vi "RTSA_FM_Demodulation.vi"() -> ()   [LabVIEW 2020]
uses:
  <vilib>/sound2/lvsound2.llb/Sound Data Format.ctl
  <vilib>/sound2/lvsound2.llb/Sampling Mode.ctl
  Controls/FIR_Config.ctl
  <vilib>/Analysis/3filter.llb/Filter Passband Type.ctl
  <vilib>/Analysis/4window.llb/windowTd.ctl
  <vilib>/Ngene/CuLab - GPU Accelerated Toolkit/Toolkit/Low_Level/Tensor_Classes/T_Children/T1D/T1D_Children/T1D_SGL/Pull.vi
  <vilib>/Ngene/CuLab - GPU Accelerated Toolkit/Toolkit/Low_Level/Tensor_Classes/T_Children/T2D/T2D_Children/T2D_I16/Pull.vi
  3a16d78b-71d0-4033-90dd-1ad3df79cfc2.vi
  0dbdd736-41c7-4217-8948-0a4463f0bf22.vi
  <vilib>/Ngene/CuLab - GPU Accelerated Toolkit/Toolkit/Low_Level/GPU_Wrapper/cudart/Memory/PULL/1D/cudart_PULL_Data(SGL_1D).vi
  <vilib>/Ngene/CuLab - GPU Accelerated Toolkit/Toolkit/Low_Level/GPU_Wrapper/cudart/Memory/PULL/2D/cudart_PULL_Data(I16_2D).vi
  <extravilib>/ChannelInstances/High Speed Stream-c(dbl,a[.](i8))/_Read For Replicate.vi
  <extravilib>/ChannelInstances/High Speed Stream-a[.](sgl)/_Read For Replicate.vi
  <vilib>/Ngene/CuLab - GPU Accelerated Toolkit/Toolkit/Low_Level/Tensor_Classes/T_Children/T1D/T1D_Children/T1D_I8/T1D_I8.lvclass
  C:/Program Files/National Instruments/LabVIEW 2020/vi.lib/Ngene/CuLab - GPU Accelerated Toolkit/Toolkit/Low_Level/Tensor_Classes/T_Children/T1D/T1D.lvclass
  <vilib>/Ngene/CuLab - GPU Accelerated Toolkit/Toolkit/Low_Level/Tensor_Classes/T_Children/T1D/T1D_Children/T1D_SGL/T1D_SGL.lvclass
  C:/Program Files/National Instruments/LabVIEW 2020/vi.lib/Ngene/CuLab - GPU Accelerated Toolkit/Toolkit/Low_Level/Tensor_Classes/Tensor.lvclass
  <vilib>/Ngene/CuLab - GPU Accelerated Toolkit/Toolkit/Low_Level/Tensor_Classes/T_Children/T2D/T2D_Children/T2D_I16/T2D_I16.lvclass
  C:/Program Files/National Instruments/LabVIEW 2020/vi.lib/Ngene/CuLab - GPU Accelerated Toolkit/Toolkit/Low_Level/Tensor_Classes/T_Children/T2D/T2D.lvclass
  <extravilib>/ChannelInstances/High Speed Stream-c(dbl,a[.](i8))/Instantiate.vi
  <extravilib>/ChannelInstances/High Speed Stream-a[.](sgl)/Instantiate.vi
  <extravilib>/ChannelInstances/High Speed Stream-a[.](sgl)/)Channel.vi
  <extravilib>/ChannelInstances/High Speed Stream-a[.](sgl)/Abort Signal/Init Signal.vi
  <vilib>/sound2/lvsound2.llb/Sound Output Write (DBL Single).vi
  <vilib>/sound2/lvsound2.llb/Sound Output Set Volume (Single).vi
  <extravilib>/ChannelInstances/High Speed Stream-c(dbl,a[.](i8))/)Channel.vi
  <extravilib>/ChannelInstances/High Speed Stream-c(dbl,a[.](i8))/Abort Signal/Init Signal.vi
  <vilib>/Ngene/CuLab - GPU Accelerated Toolkit/Toolkit/Low_Level/Tensor_Classes/T_Children/T1D/T1D_Children/T1D_I8/Push.vi
  <vilib>/Ngene/CuLab - GPU Accelerated Toolkit/Toolkit/API/Numeric/Complex  (API)/Interleaved to Complex/T1D/CU_Interleaved_To_Complex_T1D_CSG.vi
  <vilib>/Ngene/CuLab - GPU Accelerated Toolkit/Toolkit/API/Numeric/Multiply/T1D/CU_MultiplyC_T1D_CSG.vi
  <vilib>/Ngene/CuLab - GPU Accelerated Toolkit/Toolkit/API/Signal Processing/Signal Operation/Digital Down Conversion/CU_Digital_Down_Conversion_T1D_CSG.vi
  <vilib>/Ngene/CuLab - GPU Accelerated Toolkit/Toolkit/API/Signal Processing/Signal Operation/FIR Filter/T1D/CU_FIR_Filter_T1D_CSG.vi
  <vilib>/Ngene/CuLab - GPU Accelerated Toolkit/Toolkit/API/Signal Processing/Signal Operation/Rational Resample/T1D/CU_Rational_Resample_T1D_SGL.vi
  <vilib>/Ngene/CuLab - GPU Accelerated Toolkit/Toolkit/API/Signal Processing/Signal Operation/FIR Filter/T1D/CU_FIR_Filter_T1D_SGL.vi
  <vilib>/Ngene/CuLab - GPU Accelerated Toolkit/Toolkit/Low_Level/Checkers/Check_Tensor_Ref.vi
  <vilib>/Ngene/CuLab - GPU Accelerated Toolkit/Toolkit/Low_Level/Tensor_Classes/Property/Get_Mem_Desc.vi
  <vilib>/Ngene/CuLab - GPU Accelerated Toolkit/Toolkit/Low_Level/Tensor_Classes/T_Children/T1D/Property/Get_Dims.vi
  <vilib>/Ngene/CuLab - GPU Accelerated Toolkit/Toolkit/Low_Level/GPU_Wrapper/cudart/Memory/Utils/cudart_get_type_size(inBytes).vi
  <vilib>/Ngene/CuLab - GPU Accelerated Toolkit/Toolkit/Low_Level/GPU_Wrapper/cudart/cudart_get_Error_String.vi
  <vilib>/Ngene/CuLab - GPU Accelerated Toolkit/Toolkit/Low_Level/Tensor_Classes/T_Children/T2D/Property/Get_Dims.vi
  <vilib>/Analysis/3filter.llb/FIR Filter (CDB).vi
  <vilib>/Analysis/2dsp.llb/Rational Resample (single channel, DBL).vi
  <vilib>/Analysis/3filter.llb/FIR Filter (DBL).vi
  <vilib>/Ngene/CuLab - GPU Accelerated Toolkit/Toolkit/CuLab.lvlib
  <vilib>/ptbypt/NI_PtbyPt.lvlib
  <vilib>/Analysis/NI_AALBase.lvlib
  <vilib>/Analysis/NI_AALPro.lvlib
  <extravilib>/ChannelInstances/High Speed Stream-a[.](sgl).lvlib
  <extravilib>/ChannelInstances/High Speed Stream-c(dbl,a[.](i8)).lvlib
  C:/Program Files/National Instruments/LabVIEW 2020/vi.lib/Ngene/CuLab - GPU Accelerated Toolkit/Toolkit/Low_Level/Tensor_Classes/T_Children/T1D/T1D_Children/T1D_I8/T1D_I8.lvclass
panel:
  out "TO2":bool
  in  "Volume":dbl(slide)=50.442477876106196 scale=0.0..100.0
  out "TO1":bool
  in  "En FIR1":bool=TRUE
  in  "En FIR 2":bool
  out "GPU Model":string="NVIDIA GeForce RTX 2060"
  in  "Device":enum16{"CPU", "GPU"}(ring)=enum."GPU"
  in  "Monitor Spectrum?":bool=TRUE
  out "Processing Time":dbl=0.0026387559999420775 format="%#_3ps"
  in  "Tab Control":enum32{"Display", "Config"}(tab)
  out "Tuning Frequency":dbl=94700000.0 format="%#_4pHz"
  out "Input Spectrum @40MSa/s":sgl[](graph)=[-195.74269, -189.41739, -197.96577, -186.8748, -177.78354, -207.19247, -210.08214, -169.48285, -199.98706, -181.2713, -191.27261, -190.39642, -183.04224, -200.49988, -182.10933, -202.1692, -171.8974, -212.6142, -198.6505, -188.77963, -196.58716, -185.11966, -179.15524, -201.63844, -186.4834, -200.24901, -200.46278, -185.01138, -196.53717, -185.41953, -188.2061, -197.32983, -198.37976, -189.08173, -186.4801, -201.58752, -183.60147, -196.62645, -209.84062, -175.21713, -201.1939, -183.62234, -188.5773, -194.54077, -187.52832, -196.452, -179.08649, -209.40384, -163.16777, -216.1494, -188.34988, -194.7367, -193.2518, -188.87604, -181.25575, -185.2676, -205.463, -175.0271, -189.99478, -185.21825, -217.7869, -148.38145, -186.99852, -193.43365, -184.94409, -196.96593, -200.83698, -179.0772, -158.98729, -196.02713, -186.37502, -190.57826, -179.79578, -201.81923, -197.45091, -148.32356, -192.8893, -191.20778, -174.6517, -207.94998, -203.33885, -161.64241, -131.68286, -220.83685, -200.93349, -174.15923, -180.49594, -188.55728, -148.40103, -184.10155, -186.05206, -187.3106, -195.83875, -181.08089, -202.82848, -138.07559, -196.52895, -186.6818, -190.37135, -186.28654, -184.90488, -201.55486, -138.26837, -210.65378, -183.64981, -195.04991, -194.87773, -182.96739, -198.64731, -153.37822, -174.90775, -199.01616, -211.22891, -164.32329, -217.64474, -139.66325, -199.33466, -174.90346, -182.80539, -190.15744, -189.8559, -187.95468, -148.82297, -208.66429, -182.54468, -194.26491, -184.6078, -193.6792, -197.16394, -171.52176, -187.44923, -194.2014, -204.48964, -171.77802, -190.1632, -186.1087, -182.00583, -195.08395, -181.37729, -190.31065, -191.36617, -178.82884, -185.42416, -187.32373, -200.90483, -176.50023, -210.23215, -166.6416, -203.82146, -172.44035, -187.1689, -190.90376, -192.03012, -183.53299, -157.26236, -207.40034, -161.06886, -210.72063, -176.25487, -202.25426, -186.92038, -191.53656, -169.67162, -201.85265, -186.35945, -190.17638, -212.25063, -158.53001, -197.0443, -169.26753, -187.78165, -187.05241, -186.73935, -190.46033, -165.65817, -206.38417, -170.5293, -200.23378, -183.6117, -188.53166, -181.8641, -196.68568, -199.11188, -176.69498, -195.53632, -177.91652, -173.9989, -199.72652, -180.88602, -195.96918, -200.19397, -180.98767, -193.51463, -184.69269, -188.42079, -189.31044, -189.34908, -164.00891, -188.15671, -187.6685, -208.48935, -156.22752, -187.80191, -195.10979, -213.33582, -166.73424, -195.67708, -179.99205, -147.39429, -209.93341, -177.22604, -194.27255, -194.939, -177.47406, -183.4195, -169.53806, -174.64153, -205.40869, -204.04027, -170.66547, -210.51685, -137.90729, -209.49599, -159.64774, -187.99612, -180.23668, -184.443, -194.431, -156.34924, -188.06058, -174.99947, -197.48386, -177.35445, -202.9296, -172.40001, -138.24834, -194.16797, -174.40512, -177.88834, -197.96823, -195.09995, -172.943, -141.90923, -217.37851, -169.23444, -211.18329, -200.83621, -175.99387, -170.27701, -178.55672, -187.83878, -182.21503, -186.92697, -181.6316, -213.66022, -135.03447, -191.48155, -184.64091, -193.85176, -187.58223, -175.6016, -196.7725, -142.11462, -213.91203, -190.64478, -189.34833, -155.91429, -215.54855, -185.00414, -174.82974, -198.02411, -178.01585, -175.61082, -193.04663, -213.31558, -159.08774, -190.12689, -186.42654, -181.06842, -192.70415, -155.9604, -213.46754, -180.3043, -195.27753, -199.19534, -173.43048, -193.90578, -181.99883, -189.78079, -185.80624, -190.17441, -184.62546, -182.52776, -194.55115, -184.50815, -190.79994, -160.68762, -215.37553, -197.46634, -181.3955, -177.1972, -200.45686, -176.51576, -191.98735, -182.32144, -189.93591, -190.15572, -184.90158, -203.78175, -160.18504, -192.09804, -184.6589, -207.59732, -167.4255, -172.29324, -198.27101, -156.70982, -212.14087, -174.07478, -204.68452, -196.18216, -184.15126, -179.11469, -192.19492, -182.80566, -192.27586, -199.1782, -173.42554, -200.50093, -171.43391, -199.34888, -177.22455, -190.31883, -179.93446, -186.94725, -193.47482, -179.09152, -196.70901, -190.80215, -185.04414, -190.51924, -188.849, -187.51125, -188.1037, -198.79588, -176.79057, -182.37628, -191.82182, -199.02907, -180.57051, -178.42291, -197.43909, -197.14944, -184.18706, -193.50587, -181.35849, -193.85284, -184.74783, -196.14502, -177.94083, -175.58768, -199.3913, -205.84045, -166.62898, -182.3001, -189.97084, -205.98883, -173.449, -154.80365, -218.56387, -199.15924, -180.85127, -187.6759, -189.15338, -185.8471, -188.48358, -169.62534, -202.81235, -197.51581, -179.65427, -202.01872, -175.79327, -183.49405, -193.51822, -177.77408, -198.46655, -193.52657, -180.05128, -198.38701, -177.78926, -182.94539, -195.77693, -184.131, -190.12482, -189.75867, -186.28546, -178.21646, -194.27655, -196.67021, -178.86597, -189.16808, -186.85674, -184.6819, -190.5583, -167.67056, -211.32664, -203.6424, -180.19235, -191.418, -190.6315, -176.37115, -201.9509, -191.95174, -185.47487, -201.02167, -177.16771, -169.40616, -165.02852, -192.35905, -183.64273, -181.81003, -202.13568, -196.17786, -185.08281, -200.75507, -181.38513, -190.1604, -189.65894, -211.30966, -168.3715, -185.54094, -189.09674, -182.38963, -197.77698, -181.56042, -197.46268, -195.4049, -182.81494, -194.85782, -184.77666, -190.93517, -186.70856, -193.27486, -181.2706, -173.21059, -202.30948, -185.96179, -197.89378, -186.83722, -191.67705, -183.90948, -193.72458, -188.30635, -189.82983, -197.59773, -180.55821, -199.9292, -182.10416, -182.00824, -191.77815, -189.35411, -187.07283, -180.2724, -191.99635, -176.05211, -201.34453, -179.73532, -198.52907, -197.54073, -178.97781, -205.81781, -176.04134, -175.11928, -199.26859, -190.16522, -188.51375, -187.94183, -192.84685, -193.45308, -187.01357, -193.08618, -180.87343, -205.31615, -179.09709, -188.41919, -191.88397, -192.83151, -184.4772, -183.84546, -191.43561, -195.08356, -187.77808, -187.4573, -190.17656, -184.23997, -193.37164, -196.05486, -182.97864, -181.55864, -195.7385, -183.38776, -192.6819, -196.89012, -182.30302, -195.18745, -184.68489, -176.64151, -200.95445, -182.89645, -198.37308, -181.76396, -194.17067, -197.69849, -179.75114, -188.21004, -189.08728, -193.60905, -186.89734, -202.16547, -177.92674, -196.88776, -184.23666, -185.79996, -194.05707, -190.98181, -186.4907, -191.83917, -185.33795, -169.80353, -205.77771, -203.49355, -180.60364, -192.09518, -183.0747, -183.6839, -193.47853, -182.59251, -200.16666, -196.46454, -184.5156, -188.73198, -190.97389, -183.13387, -193.04475, -177.49374, -206.70563, -180.98363, -195.24359, -173.97331, -206.24709, -181.13123, -195.54118, -185.35872, -197.09697, -193.22803, -182.22028, -183.23901, -196.27748, -182.29858, -198.15428, -175.53256, -198.99547, -173.92096, -198.77425, -197.84251, -177.60735, -195.11566, -189.01703, -193.99232, -185.8124, -187.33467, -193.51767, -201.58257, -178.17609, -199.5869, -177.50882, -203.84482, -176.02805, -190.78548, -185.5587, -172.602, -202.0326, -184.32765, -199.0357, -182.5315, -192.41716, -187.35988, -190.51581, -205.80173, -172.18991, -188.78091, -187.16411, -190.11539, -187.93852, -187.1539, -189.2002, -195.13934, -184.82574, -187.00949, -189.42319, -173.2787, -204.902, -181.12907, -195.47665, -168.75006, -199.82248, -191.4674, -185.42943, -188.17245, -189.06744, -199.53183, -182.90576, -198.11316, -160.85342, -180.14671, -199.02676, -184.9214, -191.0759, -180.35664, -199.8089, -180.81038, -198.11066, -190.71962, -184.92918, -197.43736, -181.45985, -193.55807, -186.31467, -182.34052, -192.68463, -204.70094, -173.932, -190.01054, -190.09348, -185.64122, -191.84073, -194.88971, -185.01176, -204.26747, -173.8661, -183.47838, -195.37393, -199.632, -181.18472, -193.18187, -188.64862, -181.03978, -203.92522, -197.75674, -176.95512, -182.28564, -199.4263, -181.7733, -193.06926, -186.10127, -192.86807, -188.24185, -192.64949, -186.85042, -191.45233, -188.1533, -187.04794, -196.27754, -178.00586, -185.0148, -193.76697, -179.6086, -199.15726, -194.98482, -179.83043, -187.9956, -187.87338, -193.78581, -187.05019, -199.04453, -178.461, -202.52354, -174.26009, -190.30734, -189.34105, -183.78018, -194.36803, -188.22824, -190.7067, -185.51607, -196.02736, -200.75928, -180.46822, -183.4245, -197.96936, -190.15611, -187.70609, -173.8864, -200.875, -182.28625, -196.80774, -190.2034, -183.7188, -206.81586, -173.97507, -194.90816, -180.9974, -195.8027, -188.61374, -196.14671, -179.60641, -185.17935, -194.00935, -200.02197, -179.20078, -195.40349, -184.52821, -187.95316, -189.6215, -200.06631, -175.73932, -176.89177, -202.82457, -165.518, -208.46895, -181.04626, -193.44891, -193.85117, -185.3646, -186.6543, -187.90628, -200.25139, -178.63435, -195.35832, -187.60956, -190.73076, -188.06755, -188.58534, -185.92862, -182.92027, -191.22156, -174.74142, -168.84543, -156.63916, -219.70845, -176.13878, -204.06227, -177.81117, -201.76746, -201.7822, -178.43472, -187.52634, -190.35242, -193.57916, -184.91158, -193.79677, -184.0501, -189.438, -185.66956, -172.68524, -204.68047, -174.7539, -197.45238, -194.46152, -181.81017, -181.06403, -203.43668, -178.02272, -204.37819, -205.87865, -172.57591, -198.11856, -179.3328, -184.07027, -195.473, -184.0793, -193.39273, -181.32649, -201.80507, -202.80008, -179.31546, -190.751, -190.08286, -178.90631, -198.46863, -179.13992, -202.45158, -181.15456, -195.50711, -181.65334, -198.9499, -196.75423, -177.41568, -184.09218, -196.51823, -195.56139, -182.33841, -169.68529, -213.48372, -190.75543, -176.25224, -189.77385, -187.66032, -197.63641, -175.45026, -187.2116, -187.70589, -204.29541, -172.36438, -195.73282, -182.71597, -193.92802, -180.95282, -181.71059, -195.70113, -200.83311, -175.2886, -188.68146, -189.48265, -221.16615, -134.66907, -184.07747, -188.84865, -219.33916, -158.58162, -195.72296, -183.64948, -213.85654, -165.40514, -172.42671, -208.80087, -179.65985, -196.88214, -168.87129, -210.16206, -194.44421, -184.70941, -172.07692, -200.18787, -186.44586, -192.07576, -170.8601, -206.91946, -183.01848, -199.70866, -202.31969, -172.91418, -214.8187, -156.60918, -175.93709, -202.24197, -178.65341, -202.66414, -182.45435, -192.61514, -189.60153, -194.88177, -159.21385, -212.41748, -201.24258, -178.97275, -158.50516, -198.59991, -190.04456, -195.08519, -189.10542, -185.90274, -206.62212, -174.01218, -179.12247, -200.17075, -191.81139, -183.9768, -188.99196, -116.071846, -193.03065, -187.32253, -188.1505, -189.24573, -198.40271, -173.25592, -173.8607, -203.36398, -172.85126, -207.7845, -189.62347, -185.80504, -184.40134, -191.04247, -192.47604, -186.80678, -183.75064, -191.99292, -194.93437, -184.38759, -189.45818, -188.36722, -186.12215, -188.8237, -171.57376, -204.75192, -186.08063, -192.89859, -195.80446, -184.2932, -183.09113, -199.03043, -180.27594, -196.4002, -194.46432, -185.47427, -181.30208, -200.32756, -197.71283, -182.0533, -175.95335, -203.46573, -212.3375, -161.08557, -193.06406, -184.25032, -181.67561, -198.72952, -203.82372, -178.9402, -173.13809, -203.88965, -192.99118, -184.69838, -185.89053, -196.26173, -195.37593, -188.56877, -193.15527, -157.78581, -175.63857, -203.62471, -217.28748, -155.526, -184.01773, -202.41327, -196.23997, -182.78207, -186.66817, -191.0715, -186.78705, -189.42276, -199.439, -179.60405, -200.62788, -179.64035, -187.37566, -190.89505, -191.33029, -192.55342, -191.54913, -185.16203, -176.74062, -203.47412, -177.35779, -201.89328, -172.91734, -204.83821, -201.5037, -119.526276, -147.87367, -220.25966, -187.16267, -190.23843, -157.32968, -218.87698, -190.16486, -189.78754, -183.16563, -193.55458, -197.09695, -185.5817, -180.56798, -200.32106, -185.34517, -187.69019, -191.45802, -190.40083, -178.74986, -197.48917, -153.5871, -214.1705, -183.34412, -200.63457, -176.47627, -202.46004, -194.18771, -187.68317, -191.54227, -189.70715, -188.59653, -191.87093, -173.11081, -206.3548, -180.87302, -190.99963, -191.0769, -188.76279, -190.04332, -193.119, -183.89044, -188.12209, -193.84462, -187.92197, -179.32776, -200.28671, -204.97983, -171.66426, -198.12114, -180.73933, -188.5141, -192.52977, -205.67099, -174.43037, -208.18336, -174.00475, -186.52412, -195.2379, -186.84808, -190.1786, -190.19687, -189.23727, -208.80399, -155.42078, -207.51308, -179.38536, -189.53627, -186.35168, -193.16061, -159.78076, -212.83939, -146.18219, -200.63477, -184.47049, -200.62979, -177.1814, -200.16962, -176.87411, -185.30708, -197.40443, -191.62248, -171.82266, -189.8419, -188.18628, -197.6218, -180.62967, -175.76228, -208.78006, -200.99417, -180.41394, -199.3006, -181.72798, -201.12634, -173.13852, -166.58553, -206.70534, -221.22916, -148.7924, -189.16725, -188.79414, -212.59601, -157.398, -186.45464, -194.56696, -196.86357, -180.91273, -193.42668, -182.73383, -192.90036, -185.88786, -202.79568, -177.44011, -197.36086, -182.63985, -193.5068, -183.40247, -189.88004, -186.20396, -157.93169, -217.3342, -186.47325, -190.21826, -163.80817, -212.45142, -167.32716, -205.21638, -184.1956, -198.29587, -183.30295, -195.5156, -194.17276, -187.58098, -194.94264, -190.65816, -199.07474, -177.49187, -187.11874, -197.44623, -166.58891, -206.83578, -196.70804, -183.52089, -157.26619, -218.8223, -200.62996, -174.35234, -184.57187, -191.47333, -195.07039, -186.07417, -170.97934, -204.33018, -154.83844, -214.213, -179.66026, -203.34221, -196.78896, -181.68123, -174.27478, -178.68973, -197.06683, -181.99005, -186.50429, -171.16731, -192.04079, -185.74586, -184.13614, -184.67624, -185.24327, -191.98592, -165.53426, -203.41803, -181.38786, -196.78717, -175.52249, -191.34558, -212.19786, -171.84474, -183.61748, -159.76216, -195.22023, -186.26144, -174.94064, -186.22449, -194.4982, -182.47023, -170.46233, -194.40005, -178.8011, -201.4556, -199.1283, -157.98419, -183.19116, -193.48149, -198.69939, -166.50403, -172.8824, -206.6117, -210.34903, -134.90779, -184.22588, -194.88435, -207.4565, -162.76822, -180.67319, -198.89256, -198.71794, -163.78294, -185.27856, -191.23282, -219.17374, -146.33923, -192.4475, -191.27649, -212.21582, -149.86374, -188.51135, -193.20216, -225.62909, -131.90126, -192.3782, -187.9991, -207.94868, -168.3385, -174.84134, -202.43971, -191.78278, -191.43015, -184.97823, -194.87613, -208.24762, -167.42395, -185.74971, -196.90337, -194.10152, -186.6922, -150.13821, -219.32994, -183.80692, -196.43405, -142.83241, -223.45161, -178.8495, -198.8822, -184.22342, -192.63425, -209.07336, -172.54628, -192.61403, -190.15865, -206.83885, -180.77411, -184.27255, -193.14558, -181.46156, -195.76619, -153.32103, -210.33577, -179.42393, -201.40341, -156.85504, -211.7409, -179.98999, -201.5816, -172.84366, -200.81168, -196.18047, -182.20297, -181.28857, -196.08066, -193.403, -192.20592, -177.35182, -201.54605, -188.62921, -189.99376, -170.15437, -188.86877, -185.97147, -189.24573, -186.8281, -180.4254, -191.06854, -188.97643, -172.47276, -203.20766, -188.69632, -191.39883, -193.95235, -183.7786, -177.30202, -196.47171, -212.84901, -170.49394, -189.82143, -198.14185, -173.23187, -186.07458, -178.18758, -196.65565, -198.92278, -172.43433, -176.86655, -206.37057, -204.0325, -174.2856, -178.89056, -200.70874, -205.77446, -170.08289, -192.64613, -187.56111, -193.69315, -185.5565, -201.63037, -183.53497, -211.8558, -166.74493, -181.79938, -204.1626, -201.88667, -176.50552, -205.69742, -175.65648, -194.78265, -180.63756, -189.3867, -188.70036, -202.23776, -184.94876, -180.82863, -197.73401, -181.19171, -198.5386, -191.97874, -193.94275, -207.53873, -173.82608, -195.32172, -186.16954, -186.9905, -197.65956, -186.21466, -192.36447, -183.81209, -195.99075, -197.68747, -184.02963, -196.49875, -185.10973, -179.8626, -195.59015, -188.56242, -194.80621, -186.03514, -196.95006, -185.30586, -196.41934, -164.59143, -208.04025, -192.45319, -191.78305, -190.58415, -188.53743, -193.07716, -187.30292, -197.25175, -184.39612, -175.61386, -204.23521, -199.43784, -181.03302, -185.24043, -200.65685, -182.1686, -195.83627, -189.18022, -189.49529, -170.95526, -202.83437, -195.88118, -186.17946, -190.91861, -186.46317, -184.43346, -193.92728, -184.13371, -197.77502, -206.11702, -176.5531, -185.72919, -192.75739, -196.19687, -182.04205, -193.33751, -186.89597, -183.94743, -196.86421, -191.05258, -191.21733, -186.41937, -192.43243, -188.4, -195.39008, -186.8104, -190.64067, -202.90332, -179.43935, -201.4969, -181.38011, -190.87094, -193.7811, -178.1558, -205.66565, -195.48685, -187.80798, -196.51442, -190.39993, -194.1866, -190.12558, -186.25838, -195.62704, -189.98575, -191.95999, -177.2827, -201.89694, -190.32909, -191.0968, -196.24844, -181.528, -189.43227, -190.52727, -199.29251, -184.88248, -194.67467, -188.63269, -204.50865, -181.90704, -187.4264, -195.8943, -185.8627, -196.38968, -197.81587, -186.42258, -195.38014, -189.03009, -195.24983, -188.59319, -184.34679, -199.03888, -196.78711, -182.95242, -189.0618, -190.69598, -188.72232, -190.91525, -180.64314, -198.21971, -192.59349, -193.6957, -193.3695, -192.69806, -192.24278, -185.80084, -190.69757, -185.63031, -187.3471, -194.2683, -179.144, -203.736, -189.11934, -193.1881, -169.80656, -212.33641, -198.25906, -179.86642, -182.50505, -198.549, -175.88512, -204.16112, -202.05042, -180.45929, -180.46248, -199.92336, -198.2648, -154.28886, -185.95592, -195.26149, -187.04263, -193.7444, -196.79745, -184.87268, -192.07251, -190.5974, -197.79843, -183.18181, -176.69234, -200.46144, -176.40596, -203.89859, -188.24394, -193.00882, -195.8228, -181.43294, -197.5233, -183.80179, -190.46881, -191.83582, -199.98096, -184.29997, -177.78635, -203.93663, -192.68687, -188.1834, -184.62112, -198.81805, -189.32622, -194.13055, -190.88242, -186.10585, -205.6476, -177.03207, -202.48047, -177.30258, -197.25871, -186.13913, -204.76535, -177.05472, -190.97218, -190.8916, -190.91135, -189.81273, -195.63383, -187.68927, -197.80731, -186.56506, -172.47256, -208.83443, -193.57835, -191.00958, -184.66444, -193.9222, -187.43654, -191.30951, -201.79431, -181.55412, -177.32756, -206.89374, -188.3987, -188.98311, -200.8731, -183.91905, -182.70123, -198.05968, -188.36333, -192.76967, -186.72423, -195.98213, -186.45798, -193.47632, -192.84338, -185.53712, -189.35327, -190.85669, -185.8429, -196.71185, -191.08325, -191.96945, -188.23274, -194.45145, -185.44861, -200.02235, -187.22798, -193.94647, -201.80418, -182.79211, -184.70044, -196.89684, -195.55502, -182.7244, -208.56331, -162.95026, -187.378, -172.60947, -187.9456, -152.14302, -176.35599, -138.89725, -155.2241, -181.32605, -164.7741, -199.91524, -184.2147, -188.90556, -193.44952, -182.77026, -193.00357, -191.02682, -203.3522, -177.02792, -191.85779, -193.42738, -199.22925, -183.06975, -195.23166, -186.97427, -184.8055, -204.04184, -199.53363, -182.12762, -195.76491, -185.3503, -198.1117, -184.2038, -186.57253, -198.38815, -186.23529, -196.91286, -193.22092, -187.2376, -205.8896, -178.20949, -167.4064, -208.84552, -195.07605, -185.55374, -180.05014, -201.31519, -196.44177, -186.3424, -191.94278, -192.74124, -197.46384, -185.61827, -187.85521, -192.14662, -177.94951, -203.15175, -187.03029, -196.73993, -186.73123, -195.45041, -193.79988, -184.8662, -178.5177, -204.0437, -200.95734, -179.59984, -183.99051, -193.41261, -199.99857, -184.68716, -188.79532, -194.2049, -184.0103, -193.80045, -209.47162, -173.62518, -186.41495, -193.8479, -184.3659, -197.20934, -182.40048, -197.04053, -183.3949, -201.5119, -197.21918, -182.39781, -197.1912, -191.04408, -187.81377, -197.64705, -191.97954, -190.81319, -190.42664, -190.25313, -175.40588, -202.52274, -194.7638, -186.11673, -177.4515, -202.72772, -184.06903, -198.07481, -216.20436, -152.06027, -191.1452, -193.58553, -187.03975, -194.24889, -188.26553, -193.80511, -206.30894, -172.91588, -198.21024, -186.64241, -189.6189, -188.55128, -191.66002, -191.63033, -188.4096, -194.137, -189.89308, -193.85898, -182.1131, -202.55423, -201.83742, -185.42441, -177.77771, -201.0381, -196.26547, -183.61444, -187.01328, -196.59454, -200.1443, -179.01787, -189.74231, -193.78674, -202.45541, -181.19833, -196.34738, -184.66475, -216.95268, -159.18626, -197.28897, -137.86087, -155.2312, -133.27106, -166.67075, -168.11159, -179.91257, -197.84956, -189.98523, -190.43866, -196.80594, -186.84445, -201.60715, -181.66486, -181.23363, -199.91142, -187.22119, -192.94858, -188.41643, -198.44666, -174.0528, -204.65596, -194.36688, -185.94765, -180.58508, -200.75227, -193.44684, -184.98016, -173.87839, -203.89015, -186.15773, -198.88802, -178.21936, -205.4107, -185.48743, -194.61043, -195.39603, -185.37846, -191.21773, -188.10925, -200.3039, -180.20209, -190.82053, -187.56538, -188.32278, -189.20177, -188.77043, -196.83548, -184.97852, -198.64398, -186.05264, -192.88943, -203.09776, -173.39952, -197.70993, -184.57762, -185.0474, -203.53333, -186.3528, -193.89603, -188.58934, -194.36415, -190.86581, -193.89468, -186.70177, -200.33531, -204.98097, -177.44777, -190.53375, -188.11224, -206.1929, -175.97458, -194.14935, -186.17178, -187.1023, -197.19373, -187.74547, -194.22394, -182.99411, -200.57779, -189.01733, -191.59714, -189.40321, -190.77592, -190.85818, -188.64459, -203.61134, -174.22845, -197.33759, -171.14072, -165.13416, -202.61336, -187.1763, -193.81345, -205.43855, -159.86014, -173.34015, -165.64815, -184.49884, -142.09431, -164.26512, -137.39813, -139.75026, -156.8836, -126.72188, -181.68411, -142.50829, -199.97372, -172.51213, -199.3741, -189.83559, -187.26611, -192.27586, -190.14154, -205.53296, -158.59499, -172.43695, -188.58621, -180.36868, -175.81111, -175.68524, -182.10832, -162.84625, -202.6215, -196.59448, -185.9205, -134.09406, -215.86551, -195.77127, -187.50839, -201.7305, -185.99158, -193.07391, -186.5491, -200.79198, -182.2993, -177.49808, -204.96005, -188.1354, -195.6049, -198.26228, -182.23988, -178.47003, -197.9984, -192.83087, -189.23335, -186.22202, -197.45015, -200.5219, -183.86229, -176.25787, -209.24655, -192.07137, -193.59563, -186.91887, -195.80844, -173.77208, -205.15965, -175.97064, -207.92912, -186.67468, -199.02214, -186.49284, -191.20338, -192.24739, -188.37746, -191.615, -184.95374, -180.86768, -199.68527, -193.10196, -189.09053, -184.5502, -196.50203, -190.46869, -196.69931, -212.51213, -146.4261, -205.60059, -164.69298, -200.36578, -141.7776, -179.25252, -149.08757, -146.41902, -191.03062, -158.8023, -208.03603, -182.03232, -194.13223, -181.48787, -200.23071, -186.97227, -190.34164, -188.65941, -196.14035, -188.32098, -197.36583, -198.0842, -187.26082, -185.27336, -196.99026, -188.82722, -191.0915, -183.83293, -198.55188, -200.82872, -185.37743, -181.47913, -200.36812, -201.69925, -183.8984, -185.93506, -192.07556, -181.48116, -197.62941, -164.33006, -201.91508, -184.5673, -194.86337, -191.09584, -189.98563, -203.82101, -166.74011, -194.87782, -187.48312, -181.86546, -199.4901, -185.1796, -198.89821, -189.07292, -196.1205, -189.25865, -190.59714, -189.38431, -191.72296, -191.74872, -189.0185, -208.5624, -171.53297, -205.17606, -163.45026, -189.37111, -194.5928, -193.57152, -186.10611, -194.85631, -190.8299, -190.0316, -188.52315, -193.57135, -188.89287, -184.16045, -193.66328, -203.85384, -167.62634, -199.25159, -149.4211, -192.78207, -138.19174, -170.41202, -146.9278, -166.08737, -154.43666, -140.54112, -173.48984, -138.6968, -187.69519, -141.95038, -204.9781, -154.36826, -211.18294, -165.48547, -212.61703, -174.5232, -211.14296, -191.98743, -191.3793, -199.74654, -182.38893, -185.26163, -195.83232, -190.90244, -190.59686, -192.71648, -189.13358, -189.45816, -192.56526, -190.19307, -191.12083, -184.53131, -194.02202, -195.70529, -187.24881, -201.6894, -177.56903, -202.6443, -171.6817, -205.15704, -158.07957, -184.67035, -163.62123, -178.61148, -165.7226, -166.05177, -184.58736, -162.96959, -201.16083, -179.61914, -195.98976, -190.61215, -189.82114, -185.20534, -195.89984, -188.71272, -188.47711, -189.99379, -191.84158, -182.65181, -200.48135, -185.54607, -196.64053, -185.34772, -197.84706, -191.65512, -194.51167, -192.97427, -189.02815, -191.3264, -194.12003, -203.51999, -179.08774, -210.75607, -171.2248, -200.20807, -183.89247, -193.78604, -191.85468, -180.79564, -191.0302, -195.25621, -174.13094, -169.5726, -200.12541, -188.12827, -181.5707, -168.28313, -207.8508, -168.75317, -212.05429, -189.90417, -191.5548, -203.39682, -176.88046, -185.89575, -194.29384, -189.55992, -188.62848, -225.16313, -153.18436, -182.04915, -200.82361, -212.84048, -136.15706, -156.02231, -170.698, -171.71451, -158.31743, -155.06982, -174.84091, -139.59769, -193.47299, -189.66974, -171.64119, -193.9153, -139.95023, -165.83907, -130.07794, -160.02617, -126.101395, -158.4574, -114.84449, -123.04937, -142.46855, -130.12158, -143.1568, -123.88716, -161.23659, -120.383804, -184.07596, -131.37828, -199.8854, -164.82785, -198.31317, -198.22153, -138.6459, -183.49301, -144.96692, -164.40393, -160.86623, -160.72032, -161.41286, -135.86105, -199.2756, -189.28261, -163.53831, -165.22136, -186.00952, -184.94249, -168.59592, -159.54541, -193.76245, -200.66353, -147.1806, -197.54993, -130.82959, -164.53647, -136.67297, -162.85992, -129.16914, -151.11707, -139.9051, -149.97052, -131.84717, -121.87078, -160.8102, -138.88426, -154.63773, -130.99158, -172.31158, -126.45973, -193.18176, -154.45328, -194.26627, -201.2255, -157.28595, -175.46092, -182.79639, -174.05722, -186.00507, -173.47247, -189.58246, -155.78067, -217.1175, -169.333, -212.81529, -193.41565, -185.87537, -183.44139, -197.53038, -176.54729, -204.6188, -196.09692, -186.54742, -197.69962, -185.30354, -196.41432, -186.83072, -190.26495, -187.32596, -206.71141, -171.01451, -181.50006, -194.14456, -184.87106, -190.9832, -167.84215, -204.69208, -179.03389, -199.20193, -209.54445, -168.67534, -184.0219, -196.64197, -197.07649, -189.52426, -178.96301, -203.17392, -179.07034, -197.7478, -206.9845, -174.84883, -191.2287, -192.23456, -201.32375, -177.18625, -180.75375, -198.7896, -191.07382, -193.03215, -215.44524, -164.18694, -205.9758, -170.92082, -201.16049, -183.88504, -180.11127, -199.40846, -175.17973, -203.90657, -189.98436, -186.23004, -186.79677, -193.01949, -193.69377, -187.33417, -179.3281, -198.99397, -196.47017, -186.31245, -176.65439, -204.53793, -193.63457, -176.69127, -197.9112, -163.94456, -195.63118, -128.46931, -175.68588, -121.03154, -154.87186, -96.88803, -130.38232, -85.55119, -96.445366, -155.56584, -116.313614, -178.21706, -134.75912, -192.28706, -168.43054, -189.20746, -166.35089, -204.80707, -181.10661, -193.0843, -185.46194, -193.95714, -184.36383, -191.28407, -184.3252, -196.85173, -186.66542, -193.35919, -187.09218, -188.4535, -198.02718, -180.2515, -190.45534, -187.31592, -191.6055, -184.97583, -197.84488, -179.75603, -183.3238, -191.62306, -174.43346, -183.42989, -171.05055, -190.08809, -190.6579, -166.59595, -184.88618, -174.26276, -181.54439, -174.74121, -178.50633, -183.05229, -176.30643, -183.36708, -176.65439, -194.65648, -203.92389, -177.835, -199.10901, -174.13994, -157.28305, -190.90758, -186.31934, -193.34607, -202.25623, -172.80455, -214.8862, -136.83447, -168.37831, -164.43042, -163.72491, -167.43018, -168.42717, -162.41011, -141.37773, -197.6646, -208.71426, -133.7107, -198.5633, -135.18277, -177.81644, -120.25853, -161.04443, -110.21414, -137.06795, -113.05885, -112.28743, -127.402756, -112.125374, -138.80591, -136.38509, -124.32542, -110.7782, -175.02658, -133.79851, -192.29256, -162.71391, -189.41217, -202.9614, -142.11288, -178.90092, -150.5877, -169.8817, -158.15399, -165.8725, -162.50974, -137.63687, -204.92838, -188.15929, -186.7095, -183.18242, -194.25409, -178.20424, -191.36893, -181.12074, -190.12053, -207.07077, -158.94006, -184.50807, -182.80894, -190.94804, -176.09546, -196.89154, -177.52281, -191.01486, -176.41342, -180.16441, -170.25175, -173.03522, -192.07831, -179.39986, -184.52951, -167.78084, -201.72198, -201.28825, -159.7324, -204.28354, -163.61911, -171.14476, -200.85574, -171.0124, -196.77713, -186.86856, -184.13713, -173.21992, -188.02325, -198.8572, -173.62369, -180.52824, -188.77576, -175.40009, -193.08163, -180.89551, -194.18393, -189.88484, -180.27058, -193.11493, -172.5008, -189.37366, -166.40329, -180.86168, -174.10004, -195.30197, -147.69492, -181.8171, -149.68259, -169.82289, -156.53671, -159.54744, -172.74397, -163.68086, -182.94844, -151.9588, -205.33488, -158.95554, -206.4908, -196.42622, -166.62485, -193.35416, -178.24425, -169.15709, -202.51807, -183.65268, -184.60532, -176.11607, -194.6279, -212.08823, -152.41058, -186.33862, -171.38446, -164.67062, -191.20534, -191.23288, -163.62793, -165.4931, -198.262, -185.14261, -176.94804, -187.03734, -169.9688, -187.1225, -155.07689, -175.16058, -150.63904, -171.8685, -148.82468, -162.02252, -149.66248, -138.01904, -177.19772, -140.60704, -190.66542, -155.73741, -183.9245, -165.07217, -184.5511, -180.25511, -184.51318, -179.69807, -189.67827, -210.48276, -141.14078, -179.87488, -181.2749, -181.0631, -180.45824, -176.43758, -188.22508, -170.37477, -202.93318, -187.2042, -185.58377, -172.5014, -191.9975, -160.01414, -205.24808, -199.6875, -172.01886, -170.1298, -201.42479, -174.44067, -185.68901, -177.56474, -185.10736, -196.56685, -170.78738, -178.67484, -183.3616, -180.43149, -181.3714, -176.28006, -183.8397, -177.80862, -183.76614, -198.67375, -170.83282, -174.8118, -191.70657, -191.67416, -179.77039, -156.42699, -204.48048, -180.94664, -183.6885, -171.95378, -192.49088, -174.28357, -191.92807, -210.12195, -161.0991, -193.28629, -168.89903, -188.48003, -183.15787, -173.32515, -194.57896, -180.13933, -189.02063, -186.46074, -188.39917, -181.76436, -189.62648, -167.27913, -194.42235, -188.70982, -175.16718, -180.38287, -186.0159, -181.29898, -187.54453, -155.90543, -213.71045, -190.33505, -180.55367, -201.07281, -171.75262, -187.44191, -178.76186, -183.32274, -182.35109, -176.1148, -192.97893, -199.20126, -172.31702, -187.24084, -181.1983, -176.33904, -193.12546, -174.5784, -189.49805, -199.86734, -167.60918, -181.28194, -185.21053, -175.87582, -194.07874, -193.05917, -180.206, -191.24646, -181.69078, -182.16084, -185.80379, -173.42996, -191.35988, -185.24965, -183.2225, -205.95682, -153.71556, -194.86029, -168.46593, -192.45496, -174.90393, -177.298, -188.45526, -175.835, -195.0782, -175.67458, -189.6373, -203.04575, -139.66486, -171.38771, -145.16881, -163.63596, -137.85239, -159.53522, -140.06654, -146.22865, -143.08313, -123.52735, -176.06879, -125.90134, -183.49388, -143.43788, -183.99893, -152.50981, -199.25168, -171.58669, -191.38521, -184.62529, -183.37938, -185.77371, -180.33205, -194.0642, -169.88531, -190.36032, -168.16782, -166.00374, -195.19934, -191.39716, -178.37398, -182.95728, -187.50592, -197.02605, -172.09305, -177.59831, -187.22626, -183.65976, -186.37248, -190.33592, -181.05249, -166.59784, -182.38332, -185.84575, -169.18433, -166.26064, -185.50049, -176.50339, -172.95186, -176.5646, -176.47357, -175.93973, -182.24538, -171.21312, -180.13213, -182.97409, -188.0494, -192.7496, -172.3962, -167.19298, -205.60944, -173.6522, -198.1665, -163.78094, -199.97523, -197.52089, -170.97311, -202.97655, -160.41933, -191.97441, -176.075, -185.52492, -184.72556, -190.37292, -183.79388, -164.19073, -203.29913, -170.94289, -200.91917, -182.07005, -190.76117, -208.39665, -157.56725, -192.18848, -181.29399, -208.84943, -138.5236, -158.75172, -160.13872, -134.87772, -206.34985, -179.00684, -192.75064, -196.68402, -177.10059, -181.49849, -193.61642, -195.11887, -175.22597, -205.17055, -161.889, -177.69077, -183.56645, -174.23274, -189.88196, -172.09811, -193.05713, -177.0151, -193.54607, -169.21118, -204.61539, -177.90546, -193.59958, -178.84593, -192.75787, -199.66199, -174.02805, -198.5082, -176.43001, -209.97784, -157.26028, -193.30545, -169.05698, -177.84003, -183.89195, -166.48347, -188.7169, -174.38922, -174.5773, -170.94165, -181.01823, -156.1092, -197.27487, -167.87437, -195.56645, -174.03082, -194.88116, -213.70828, -151.99834, -197.66951, -172.23335, -188.24057, -183.20042, -186.3997, -187.25082, -180.71591, -189.07237, -174.69135, -191.21075, -161.26482, -208.35036, -188.82059, -180.81683, -202.28143, -155.91386, -188.62, -183.33675, -173.36212, -194.51566, -192.90466, -178.23914, -189.7453, -171.95924, -184.4326, -171.33157, -184.7204, -166.30756, -182.11855, -153.82892, -151.85582, -187.64627, -171.83817, -180.50739, -169.40941, -187.583, -173.5932, -185.4643, -180.04994, -183.89647, -144.83023, -213.44199, -179.44078, -195.35863, -203.32503, -164.55019, -146.54247, -207.79474, -197.00467, -166.71275, -192.36002, -171.13991, -192.88486, -170.47076, -183.3673, -182.6104, -168.34087, -189.37506, -182.07326, -183.05739, -170.60765, -196.01212, -162.8365, -199.49992, -167.37958, -193.3986, -198.11739, -166.3612, -185.2846, -179.85495, -177.82137, -187.0852, -195.24902, -170.97855, -159.62582, -199.95213, -186.68048, -175.88933, -169.50723, -197.80753, -183.15384, -185.3919, -204.4356, -161.8593, -201.90843, -160.62935, -194.74872, -166.2311, -182.70012, -178.22064, -177.04987, -193.60722, -203.34525, -162.83612, -174.73041, -188.37668, -155.15494, -207.166, -146.47983, -210.10387, -194.81604, -180.01236, -206.44247, -160.95486, -196.75673, -170.12355, -191.63449, -176.7175, -205.48586, -156.90579, -181.49109, -177.3662, -158.51009, -188.72852, -168.767, -178.39838, -148.92178, -219.52293, -193.50908, -171.31842, -206.95409, -157.7565, -190.67992, -159.12906, -184.99445, -134.59511, -176.77182, -107.293564, -126.31838, -128.9252, -111.49228, -176.51065, -140.80434, -188.24492, -151.47632, -194.54422, -196.61429, -162.1531, -204.90245, -162.09116, -189.13797, -180.6247, -178.40497, -169.3446, -165.91556, -183.4978, -161.62016, -185.65555, -162.97708, -198.11345, -194.9502, -179.29854, -171.47298, -193.40671, -146.8279, -217.9404, -183.4381, -190.97324, -196.96437, -174.01074, -194.30106, -170.72063, -172.81429, -185.11102, -186.68047, -186.00822, -173.35533, -184.59227, -175.33452, -179.33374, -174.72499, -181.7564, -205.38681, -155.54214, -179.7719, -178.21983, -160.17151, -206.69348, -179.81972, -192.02766, -164.84628, -197.9602, -180.26558, -188.74713, -162.10469, -193.18332, -195.23402, -169.74438, -152.62012, -212.32562, -185.27054, -186.17012, -214.74046, -151.16339, -188.40228, -175.81346, -169.29349, -176.84258, -183.18364, -185.91287, -196.86055, -161.60918, -180.56007, -155.9571, -158.65337, -165.62111, -177.31613, -144.47601, -173.80823, -131.11147, -145.75615, -140.8993, -134.09486, -167.77904, -133.72372, -197.64352, -163.29694, -195.96829, -180.04974, -189.77837, -181.26347, -193.36002, -167.44778, -201.7055, -157.61531, -203.4722, -207.54053, -166.22192, -189.6431, -173.46869, -187.31966, -181.0359, -180.64705, -189.6848, -181.46152, -181.09636, -183.67389, -182.91446, -174.99634, -196.4274, -151.90672, -215.50766, -193.81218, -177.52203, -205.01547, -155.52031, -184.61261, -177.32289, -180.27707, -171.99454, -164.64742, -187.92088, -169.98874, -194.96275, -168.99348, -199.20876, -158.0149, -209.00891, -180.8724, -190.75682, -213.23708, -156.30293, -173.56049, -187.06982, -197.93704, -165.01773, -191.6106, -172.98943, -185.81465, -185.70924, -172.61981, -184.55766, -176.47607, -190.85861, -169.26953, -202.39476, -148.52411, -220.25722, -209.32098, -159.02171, -188.81653, -171.0237, -212.77432, -143.78807, -183.90245, -141.68326, -180.86382, -125.96388, -150.67589, -155.1133, -132.80463, -174.67169, -146.7521, -185.56026, -150.20645, -192.11427, -173.90956, -196.59338, -203.43315, -152.0143, -182.07317, -190.39604, -174.34172, -189.05591, -182.37251, -184.95651, -176.8553, -187.51799, -163.33334, -199.67653, -175.10832, -200.45215, -173.18326, -189.55011, -193.5201, -180.13016, -207.1995, -150.54306, -177.04973, -188.39226, -202.27399, -164.60876, -187.8966, -178.36255, -191.56955, -170.95023, -197.30035, -136.3788, -156.10934, -157.96225, -137.88394, -193.48666, -173.32977, -186.3339, -201.47345, -165.49431, -198.79967, -166.84608, -200.53156, -164.23506, -187.02039, -185.6132, -149.91968, -213.14322, -191.41292, -181.45795, -154.55678, -207.22916, -187.81056, -176.38068, -211.60526, -150.7914, -186.05984, -183.82271, -191.84773, -173.41273, -162.66852, -202.08832, -164.93083, -193.51987, -182.63678, -186.11157, -165.1404, -192.29056, -183.52017, -185.55318, -156.7913, -202.4543, -200.90799, -164.4054, -195.96596, -171.69247, -173.65479, -194.01587, -178.68472, -182.41931, -180.09053, -193.35406, -174.0677, -187.93031, -188.74036, -176.92928, -149.3078, -211.89171, -213.45128, -148.56737, -201.01752, -173.0789, -198.2237, -156.76251, -175.1947, -188.76001, -185.98215, -166.92715, -183.14584, -178.67415, -170.65881, -183.86237, -196.5726, -171.79742, -158.22171, -194.52094, -199.5352, -150.28911, -188.6992, -154.54645, -182.23238, -128.07945, -147.66185, -149.14471, -148.6671, -154.96585, -142.55634, -196.28294, -141.01794, -200.1448, -176.1186, -182.00984, -149.11101, -208.2203, -208.60155, -144.27673, -173.78038, -186.35518, -196.29144, -157.384, -173.46463, -180.88284, -145.74207, -213.2825, -205.55928, -138.89316, -166.2012, -195.74736, -160.84721, -203.08444, -197.28531, -167.01068, -187.59077, -181.43341, -211.55376, -150.64516, -189.56523, -180.70361, -197.79375, -162.22937, -196.05544, -180.92673, -152.93042, -209.16757, -154.68044, -214.27591, -149.29437, -208.38728, -201.21973, -163.8682, -215.67741, -147.49844, -186.5203, -188.40642, -188.37831, -169.79898, -198.62337, -173.75804, -170.61237, -186.52283, -186.49113, -183.9868, -151.08882, -207.39589, -163.00916, -201.88483, -216.59372, -144.35703, -188.5333, -183.93262, -189.70702, -169.04745, -185.02274, -184.89725, -194.80132, -168.87155, -168.96649, -191.12067, -188.41162, -170.92798, -184.71973, -160.20627, -164.9551, -174.6491, -157.208, -186.36887, -182.67262, -168.19658, -196.41464, -155.78345, -165.683, -198.56793, -164.70842, -193.9494, -185.19403, -184.81831, -179.3915, -182.41965, -151.13136, -205.04485, -173.05757, -190.18665, -149.86208, -202.85278, -195.04004, -165.13225, -189.21771, -165.75935, -181.35405, -185.28397, -180.16873, -183.19217, -176.66908, -181.49423, -172.42885, -189.75084, -152.71123, -200.85612, -189.17252, -170.42761, -191.26938, -158.01224, -208.49442, -158.37625, -181.45103, -174.55353, -183.07338, -172.18947, -178.65282, -182.689, -170.39145, -184.52513, -163.91222, -196.14113, -174.7283, -189.01257, -143.16898, -211.02357, -194.23315, -173.50406, -195.14612, -158.60365, -174.19641, -158.03476, -167.70229, -184.44318, -174.63583, -179.75299, -182.21315, -181.4405, -163.26894, -196.23863, -143.21303, -210.31665, -200.15233, -158.19145, -203.34428, -151.83853, -189.11543, -174.632, -184.30853, -174.43855, -177.15123, -172.3206, -163.44598, -198.3093, -174.97346, -184.19594, -152.90695, -206.04686, -160.98328, -204.62808, -212.15938, -137.32753, -189.68819, -160.97287, -174.67155, -164.05847, -168.89914, -173.12576, -188.93866, -148.84315, -174.98642, -159.36711, -180.98866, -147.95108, -156.98465, -170.87733, -156.00468, -179.1182, -163.15419, -172.63322, -185.22308, -177.78125, -172.34885, -187.25516, -192.72449, -158.57356, -179.91638, -175.06541, -174.07509, -182.56006, -172.59753, -176.09239, -147.36008, -205.12953, -186.49777, -174.59178, -203.36533, -150.00285, -204.78653, -154.32323, -176.19252, -187.734, -194.23206, -166.26205, -180.49634, -174.22853, -171.10645, -187.39412, -184.96695, -177.34613, -210.42526, -134.3348, -153.64273, -179.54343, -172.49232, -160.5097, -187.78262, -153.20274, -154.8974, -188.48508, -195.34143, -160.79712, -190.43953, -141.68156, -173.66586, -133.44972, -169.08647, -118.76871, -154.84071, -120.786514, -126.72821, -136.99727, -131.97011, -140.10004, -113.40488, -166.67032, -122.36422, -174.24985, -135.92276, -186.67606, -159.97246, -184.39534, -188.17035, -152.05171, -171.47287, -165.37991, -154.31387, -179.70186, -165.70633, -175.42056, -147.59756, -200.08258, -191.85648, -172.90668, -184.70795, -167.96703, -166.04063, -181.66174, -169.97707, -191.87521, -189.46028, -176.7787, -174.22827, -185.06694, -152.56865, -199.52713, -142.3399, -210.90237, -176.72466, -183.21167, -190.7686, -172.3228, -196.39983, -161.98596, -184.27332, -168.15741, -166.56055, -192.48273, -183.72484, -182.1502, -177.05035, -182.34235, -153.10077, -197.10066, -164.04178, -185.6037, -201.16565, -142.38078, -188.66403, -144.92444, -163.20279, -152.35341, -154.17363, -177.03795, -146.73303, -190.26057, -148.45668, -207.39897, -173.94229, -193.20613, -169.4039, -196.75214, -192.39851, -161.1597, -212.57556, -145.40152, -199.67525, -162.64441, -193.21353, -175.73582, -168.41019, -200.84091, -197.11465, -159.23618, -149.96735, -199.48654, -144.65979, -211.21786, -148.87932, -209.848, -166.06993, -199.23685, -206.92534, -156.22832, -199.59076, -157.72733, -173.16742, -175.78313, -181.71983, -175.34698, -188.31049, -170.73355, -175.40009, -189.9465, -184.74484, -181.24359, -213.18718, -145.40495, -210.97722, -146.6872, -193.27478, -159.2707, -201.10045, -155.39156, -196.90741, -164.28926, -187.98004, -173.95451, -177.26627, -189.34831, -170.0609, -188.96524, -153.16678, -208.66556, -198.98834, -152.8821, -212.98633, -138.12886, -191.9775, -160.55925, -192.605, -170.31119, -195.86319, -171.97949, -190.8334, -173.58588, -178.56819, -189.97345, -185.54073, -177.23087, -148.3082, -210.88484, -178.55365, -171.63733, -209.9723, -142.29546, -196.02359, -154.64908, -196.47957, -162.944, -175.63704, -183.72517, -181.27147, -178.56685, -179.9884, -193.217, -183.01894, -182.3262, -155.28122, -204.93674, -187.4345, -167.90074, -192.76799, -158.73853, -211.18126, -143.9568, -186.52037, -168.57806, -171.74037, -182.16179, -186.92818, -163.21085, -194.7947, -144.24794, -163.4062, -157.12227, -164.77899, -158.10797, -169.70226, -145.05898, -144.1522, -172.13448, -155.20859, -160.85849, -154.63788, -160.84322, -161.76904, -161.75111, -153.30281, -188.23419, -168.055, -191.82233, -155.99352, -203.6546, -159.96509, -197.39532, -176.64864, -174.16443, -190.06052, -159.47238, -195.11269, -166.69724, -196.06982, -156.01672, -162.28853, -189.1099, -171.86627, -179.15924, -153.275, -198.97148, -171.21971, -178.25017, -164.28767, -187.53764, -174.95944, -179.22571, -210.67538, -149.38577, -198.1326, -157.79613, -188.04782, -173.24295, -182.80817, -180.97049, -167.99446, -199.73729, -165.06557, -196.35472, -169.63614, -194.145, -178.73264, -186.7725, -202.69315, -163.05634, -187.0734, -182.95152, -185.07469, -182.71638, -201.5863, -163.55852, -183.15805, -185.66733, -185.42888, -185.12476, -188.88567, -183.71378, -174.38806, -193.18837, -167.88115, -198.28204, -196.36755, -168.22058, -153.59544, -211.73141, -189.94101, -172.95526, -192.84825, -172.47719, -192.28473, -178.345, -186.06651, -182.70853, -171.3712, -196.7677, -184.03935, -181.05814, -198.3494, -172.54823, -182.5774, -181.86949, -175.58566, -188.20837, -185.86732, -175.585, -167.82414, -200.84848, -178.6556, -185.24515, -149.87329, -210.44455, -182.54626, -180.85722, -156.94226, -194.64713, -186.26619, -181.96854, -196.55534, -169.22302, -184.73834, -177.47092, -183.80403, -178.62276, -154.63551, -207.19368, -186.60687, -178.19916, -191.1567, -176.14629, -177.38315, -189.79463, -184.10652, -176.90213, -186.28969, -175.7991, -190.30319, -172.80548, -160.51979, -202.58698, -163.76913, -196.94055, -178.72171, -185.75385, -179.83765, -180.72481, -190.6138, -170.3219, -179.99344, -185.34245, -160.19305, -201.90752, -174.6812, -185.67996, -185.72903, -178.54321, -166.99188, -196.5752, -181.55412, -178.40686, -194.6219, -168.03375, -162.43388, -206.30205, -190.00978, -174.98898, -189.14507, -175.22362, -186.1386, -175.56015, -169.58511, -191.18207, -190.09277, -172.78796, -181.76817, -188.23807, -206.77841, -154.52017, -181.05455, -184.18674, -190.01707, -174.95784, -187.3789, -173.62735, -175.7543, -187.33215, -170.30228, -193.52911, -189.86621, -177.18427, -189.94135, -173.10211, -184.48564, -178.45293, -174.4916, -187.54213, -174.78712, -185.75299, -189.14873, -179.9368, -183.39311, -178.96951, -191.22307, -177.37529, -159.40916, -201.14804, -171.8213, -196.93153, -168.84314, -198.48685, -185.49614, -179.98537, -193.19037, -171.13664, -191.55333, -171.57158, -180.60757, -184.99266, -182.13326, -182.55724, -176.7121, -189.72128, -196.83891, -168.79114, -177.88275, -188.6068, -169.17047, -200.17157, -189.08174, -173.52176, -182.51175, -187.63853, -181.53632, -185.30733, -149.83337, -216.03537, -180.58252, -186.36299, -179.29805, -190.33128, -159.84201, -208.42204, -181.01894, -188.62157, -186.84451, -186.30241, -204.31165, -157.56294, -181.70248, -188.5474, -209.4515, -165.60336, -157.39249, -198.27571, -195.92554, -173.64346, -196.27563, -164.86667, -182.70901, -181.09886, -189.37735, -175.05951, -180.67632, -186.74425, -178.82263, -190.52844, -171.9604, -193.52037, -187.34758, -183.97758, -197.14294, -164.15352, -184.56947, -181.10902, -197.69635, -168.3513, -173.74641, -191.55006, -179.54422, -184.02696, -173.1256, -193.4728, -168.44739, -199.23749, -184.84225, -179.61365, -180.69664, -187.55736, -197.77876, -171.41095, -166.10533, -198.78433, -178.99202, -187.44476, -157.54552, -204.46384, -190.44293, -178.66742, -189.316, -172.41414, -199.63144, -165.15562, -181.95451, -180.7145, -167.48708, -196.95146, -181.22505, -186.3271, -190.72372, -172.52957, -194.01906, -176.45107, -174.98546, -194.53656, -177.03128, -191.01883, -198.45543, -171.29419, -172.80588, -191.8052, -183.45248, -181.41264, -199.08469, -169.8424, -177.1411, -189.94882, -200.82964, -159.35513, -163.57841, -201.8242, -178.45198, -186.08214, -185.09541, -181.58704, -170.41548, -193.98495, -159.03682, -212.39627, -180.74187, -186.2792, -182.88441, -188.16612, -177.52242, -185.35532, -181.91966, -180.64102, -178.11234, -186.20723, -181.95181, -185.00444, -183.5374, -184.74435, -187.61446, -182.63733, -174.30618, -192.15657, -181.01253, -186.79376, -177.21132, -189.39706, -174.639, -195.0888, -171.08987, -193.09462, -193.62917, -172.11697, -184.86353, -185.43678, -198.18796, -168.89127, -181.55127, -186.62024, -184.7821, -182.66504, -196.99763, -168.31987, -201.29836, -168.83449, -174.1459, -193.5522, -185.16928, -177.91249, -183.647, -183.02817, -170.46477, -196.93498, -181.11835, -187.96938, -189.31363, -177.80226, -165.67363, -202.5806, -187.67647, -179.71117, -188.5314, -181.0067, -180.16017, -189.4105, -200.73611, -160.29388, -188.13667, -181.61606, -168.96635, -195.84206, -157.6923, -206.9939, -194.1531, -175.99846, -186.58023, -176.23682, -190.0401, -181.89716, -205.77641, -157.04768, -174.75696, -196.15211, -184.23862, -192.5876, -165.59341, -199.48491, -206.92035, -158.95706, -172.1908, -194.1016, -190.51968, -184.48679, -209.27148, -157.59805, -189.73213, -185.06598, -177.84804, -198.13803, -180.03897, -193.29152, -199.51756, -172.15889, -188.06229, -190.73708, -185.30437, -190.37804, -204.66092, -163.26625, -196.79637, -179.3391, -185.36826, -186.67456, -199.32623, -146.13843, -199.70996, -174.3214, -165.9409, -205.84674, -172.12985, -197.0516, -182.84213, -193.23491, -170.7665, -211.3237, -188.75662, -183.61649, -207.05367, -174.4161, -177.35242, -196.4747, -195.4282, -182.22458, -217.86171, -157.04922, -173.92114, -201.3, -193.8848, -183.13002, -174.44342, -212.17958, -202.40276, -177.63977, -167.86856, -209.43973, -179.99098, -199.00099, -191.8933, -190.29482, -189.22128, -195.58208, -198.01575, -184.83441, -184.76135, -200.21335, -199.81747, -184.81764, -185.58853, -197.43, -195.01366, -185.53578, -196.82045, -187.5918, -176.04538, -201.86754, -196.85513, -187.3482, -193.89212, -192.19138, -197.98534, -183.31412, -196.19653, -186.53728]
  out "Audio Waveform @ 44.1KSa/s":sgl[](graph)=[0.03876629, 0.03662633, 0.046309587, 0.02397345, 0.03690331, 0.008707211, 0.016326718, 0.02278712, 0.011752514, 0.010768548, -0.011770525, 0.0035019787, -0.01711873, -0.0016571967, -0.0062672286, -0.017789206, -0.0025504448, -0.0029665467, 0.025803419, 0.008838584, 0.016913548, 0.0034561516, 0.0019896668, 0.01942563, -0.001790414, -0.0015434537, -0.028948216, -0.014849365, -0.025145985, -0.03011081, -0.011976552, -0.013615297, 0.006834325, -0.016281625, 0.0023292757, -0.008070825, -0.009166115, 0.014851982, 0.0155281285, 0.024416076, 0.0019365625, 0.026364032, 0.019885302, 0.026250089, 0.0355019, 0.020068282, 0.036181107, 0.02785353, 0.04768732, 0.035948575, 0.04046124, 0.027921172, 0.0057483707, 0.02243265, 0.005148804, 0.007690971, -0.019484818, -0.019517343, -0.012123676, -0.00718219, 0.008989088, -0.014936307, 0.008536909, -0.007822362, -0.005073121, 0.0030795299, 0.002370851, 0.006630057, -0.002408141, 0.035218976, 0.016201308, 0.022005083, 0.027699452, 0.0050648395, 0.0028496867, -0.0019447702, 0.014798585, -0.017427318, -0.0044139656, -0.0033726157, -0.010537903, 0.004123804, -0.0041721095, 0.010874608, -0.0154740345, -0.009594762, -0.030903123, -0.030344853, -0.006632364, -0.028275779, -0.01750656, -0.024361858, -0.008969024, -0.027725285, -0.024950797, -0.018912531, -0.04154008, -0.020149097, -0.03982389, -0.039983377, -0.042807307, -0.027210645, -0.023046514, -0.030079724, -0.012776552, -0.048840977, -0.028996032, -0.019876491, -0.011056121, 0.002207624, 0.012496174, 0.029381352, -0.0007160305, 0.020036805, 0.019107087, 0.02546201, 0.022165813, 0.015075103, 0.040340163, 0.023122985, 0.027886923, -0.0018030356, -0.008164136, -0.009179125, -0.007658255, 0.009977399, -0.015756004, -0.0025294507, -0.021609718, -0.016744897, -0.011602861, -0.008902034, 0.013635916, 0.0061179446, 0.015335653, -0.02334851, -0.020070089, -0.02376413, -0.031912815, -0.005407908, -0.0018550743, 0.017716438, -0.0030893967, 0.019449694, 0.018041987, -0.004475978, -0.0038682667, -0.009750015, 0.012221084, -0.0068966546, 0.0035463308, -0.0098720435, -0.010198719, 0.010631281, -0.0047921273, 0.0080829775, -0.01254832, -0.016668001, -0.04157397, -0.023645625, 0.0023531588, -0.0134908315, 0.0017232784, -0.025616826, -0.017813249, -0.0055522076, 0.0018273424, -0.018220393, -0.042045515, -0.021571826, -0.042078204, -0.025975946, -0.025077226, -0.020821385, -0.021446446, -0.021025173, 0.0033108806, -0.025418956, -0.023881495, -0.03890252, -0.034812737, -0.02693985, -0.0110560125, 0.010501976, -0.022882702, 0.012301719, 0.015077197, -0.014528819, -0.027889365, 0.003969176, 0.030850854, -0.0041433317, 0.010508084, -0.006606908, 0.006861613, 0.016545625, 0.011564074, 0.02090919, -0.0023024231, 0.009636345, 0.018956535, 0.056801252, 0.03869436, 0.01841652, 0.026463266, -0.015374045, -0.008988705, -0.009507459, -0.003482541, -0.026315643, -0.026442036, -0.010326079, -0.023327282, 0.0013352745, -0.009070355, 0.01793879, 0.015670963, -0.007406596, -0.008068459, -0.01796723, -0.019555843, -0.056822896, -0.025716629, -0.021142367, -0.020706233, -0.0025334025, 0.0011855257, 0.01907422, -0.013094898, -0.0025999004, 0.0011059261, 0.015808525, 0.01777622, -0.0019140217, 0.010814237, -0.014960312, -0.013145275, -0.036116228, -0.03165038, -0.020914648, -0.027718922, -0.022541016, -0.05186856, -0.025645355, -0.038079802, -0.052748065, -0.057932932, -0.052470654, -0.029678099, -0.04583812, -0.01864523, -0.03611985, -0.028123664, -0.005665806, 0.0029367784, 0.00819283, -0.005686598, 0.017265642, -0.01400038, -0.004819628, 0.0065399623, -0.008112699, -0.011962186, -0.023838524, 0.007832333, 0.0012514594, 0.028478423, 0.028658053, 0.011204325, 0.016915688, 0.015589234, 0.032706734, -0.0043169186, 0.014015283, 0.019560022, 0.0073318463, 0.018371465, 0.012778789, 0.018549424, -0.0012254269, 0.023597391, 0.0023645519, -0.008198278, 0.016583808, 0.012019424, 0.01907929, 0.0033746234, 0.022993488, 0.00577794, 0.010481902, 0.01738096, -0.01034351, -0.005878957, -0.028355753, -0.005591554, -0.0108984625, -0.0129376305, -0.01559185, -0.027410964, -0.012572353, -0.032702398, -0.008136054, -0.0026658927, 0.013799843, 0.015064927, 0.007801182, 0.016565299, -0.018514382, 0.006429874, 0.009157728, 0.0057695354, 0.0021601191, 0.01265654, 0.013398125, -0.033606455, -0.008325039, -0.0122031, -0.012488829, -0.0105149625, -0.008660178, 0.00310655, -0.010185034, 0.023814633, 0.016326062, 0.015824776, 0.013181153, 0.02490627, 0.03626892, 0.004105908, 0.028028699, 0.021481087, 0.016080957, 0.00957588, 0.025374478, 0.043520752, 0.03081074, 0.056120064, 0.04197948, 0.058060195, 0.047463037, 0.027711516, 0.034367375, 0.016042894, 0.018732745, 0.0048202462, 0.034884464, 0.034733605, 0.05695251, 0.08321429, 0.059992462, 0.070245095, 0.056306854, 0.073193185, 0.0595054, 0.040942658, 0.024251007, 0.010285451, 0.021208419, -0.01602844, 0.01376547, 0.02723659, 0.018134862, 0.014432779, 0.026388807, 0.05784004, 0.03714458, 0.055665962, 0.039940003, 0.033839222, 0.037603393, 0.04295143, 0.05519236, 0.023704054, 0.04271868, 0.03785747, 0.04615202, 0.053127795, 0.047680873, 0.041619685, 0.0044043637, 0.016491732, -0.0049060173, 0.0022565397, -0.0003660038, -0.010004351, 0.006722437, -0.0035386255, 0.016330393, 0.005155317, 0.03612096, 0.048749972, 0.032545943, 0.02109148, 0.00013619261, 0.018307758, -0.013054506, -0.014621955, -0.022076908, -0.026164252, -0.0113477595, -0.018506456, 8.364034e-05, -0.01442062, 0.0089313835, 0.0073707546, 0.00796642, 0.02587064, 0.0155659905, 0.02291464, -0.007520556, 0.011165351, 0.020308543, 0.04188566, 0.06571115, 0.058602538, 0.072639786, 0.058570284, 0.0872025, 0.078685224, 0.07135893, 0.07044131, 0.04757564, 0.047645416, 0.030350955, 0.04589895, 0.021624334, 0.03126966, 0.043912534, 0.021364441, 0.031281523, 0.019815382, 0.03467503, 0.022720197, 0.032619033, 0.027576953, 0.0040746676, 0.018499224, 0.0056448365, 0.021410825, 0.010557694, 0.027136384]
  out "Audio Spectrum @ 44.1KSa/s":waveform(sgl)(graph)={"t0"=timestamp(0 s since 1904-01-01), "dt"=99.77375565610859, "Y"=[-100.29174, -83.9092, -90.986565, -97.11911, -108.676865, -93.40738, -84.82773, -99.16064, -110.67501, -105.684456, -105.564476, -92.57231, -89.551094, -106.87368, -111.33073, -113.63648, -112.44526, -112.89085, -113.33606, -111.30567, -119.056244, -116.07376, -113.33159, -119.25409, -114.92926, -118.70466, -118.494354, -117.800674, -115.53282, -116.89979, -114.551094, -113.4704, -109.94893, -117.2646, -118.62463, -116.02999, -116.99271, -117.17933, -112.59845, -111.63831, -119.16267, -112.8147, -113.16793, -112.384125, -116.46279, -112.60225, -112.77696, -113.44975, -111.25706, -112.53971, -118.56484, -117.78303, -119.84663, -117.90972, -115.97258, -117.82146, -120.27365, -118.18381, -116.20108, -123.195625, -118.80826, -118.44725, -120.84695, -118.89989, -116.03186, -115.51068, -117.75097, -117.40709, -118.22103, -118.26777, -115.6847, -118.56783, -121.960075, -116.59388, -119.67984, -115.0425, -115.144875, -123.54707, -119.866325, -120.7032, -120.287025, -117.88625, -119.02498, -115.05426, -113.75466, -112.70831, -113.75563, -113.255875, -112.578094, -112.835945, -114.0467, -111.46239, -120.191284, -120.81108, -118.327126, -118.4551, -119.5832, -121.09807, -121.39242, -119.78077, -121.53607, -122.51818, -122.70885, -120.80067, -122.36576, -119.627464, -117.46074, -123.28147, -123.12495, -123.56397, -126.172455, -127.99516, -125.22244, -123.64855, -123.89941, -124.36775, -121.945984, -116.63512, -117.1527, -119.35282, -115.958755, -113.52826, -110.76646, -112.578255, -115.93194, -114.69864, -116.57742, -118.13745, -118.742355, -120.52937, -119.23253, -119.5476, -117.381226, -120.412636, -119.04145, -119.44681, -120.11902, -119.22622, -120.42728, -118.320595, -116.56838, -119.45873, -121.83742, -124.68266, -122.48579, -121.98211, -125.89626, -121.889, -126.629906, -130.17133, -132.35196, -139.80243, -147.39873, -154.65057, -167.39368, -165.94693, -165.84949, -165.65492, -167.76166, -171.59975, -166.57558, -171.0066, -173.42873, -167.90909, -168.30467, -171.81859, -168.68776, -171.68573, -180.00919, -176.39658, -173.71696, -167.31139, -167.70593, -173.29866, -169.21135, -175.93909, -177.6059, -176.4093, -175.08134, -173.03499, -178.65721, -172.57141, -172.02615, -168.12065, -171.93828, -172.83432, -173.6961, -177.26372, -168.84587, -111.58579, -99.35984, -111.364914, -170.13208, -174.69183, -170.77623, -171.29169, -178.43446, -178.72337, -175.54509, -182.63863, -178.0993, -178.08694, -183.30853, -188.7598, -187.5999, -186.23213, -189.70377, -185.81679, -191.11903, -191.47783, -191.52579, -192.75563, -193.63806, -193.03465, -191.1225, -196.75468, -194.52792, -197.06842, -195.94354, -193.19229, -194.84352]}
  out "Channel Spectrum @ 800KSa/s":cluster{dbl, dbl, "Dest out":sgl[]}(graph)={-400000.00000000006, 100.00000000000001, "Dest out"=array[8000 elements]}
  out "FM Demod. Spectrum @ 800KSa/s":waveform(sgl)(graph)={"t0"=timestamp(0 s since 1904-01-01), "dt"=100.00000000000001, "Y"=array[4000 elements]}
  out "Spectrogram @ 40MSa/s Map":i16[][](graph)
  in  "TDMS File Path":path=path "D:/Data/FM Band RFData_I8.tdms"
  out "Proc. Time":T1(graph)={"mean"=0.0026387559999420775, "Acq. Time"=0.009946542999969096, "Procesing Loop Time"=0.00994243799999822}
  in  "Disaply Every":i32=1
  in  "WaterFall Config":cluster{"History":i32, "X Resolution":i32}={"History"=100, "X Resolution"=4000} {"X Resolution" format="%.1p"}
  in  "Window":T2(ring)=enum."Hanning" caption="window"
  out "Audio Loop Time":dbl=0.009992085000012594 format="%#_3ps"
  out "File Read Time":dbl=0.0006694259999494534 format="%#_3ps"
  out "Acq. Time":dbl=0.009946628999969107 format="%#_3ps"
  out "Procesing Loop Time":dbl=0.009961239999975079 format="%#_3ps"
  in  "exp Avg":sgl=0.1
  out "Sample Rate":dbl=40000000.0 format="%#_6p"
  in  "Freq Offset":sgl(slide)=-20700.0 scale=-200000.0..200000.0 scale format="%08.3p"
  out "Acq. Size (Samples)":i64=400000 format="%.0p"
  out "Proc Iterations":i32=2778
  in  "stop":bool
  in  "Acq. Time":dbl=0.01 format="%#_6ps"
  # "Real-Time RF Signal Processing on GPU with LabVIEW\nSpectrum_Monitoring, DDC & FM Demodulation"
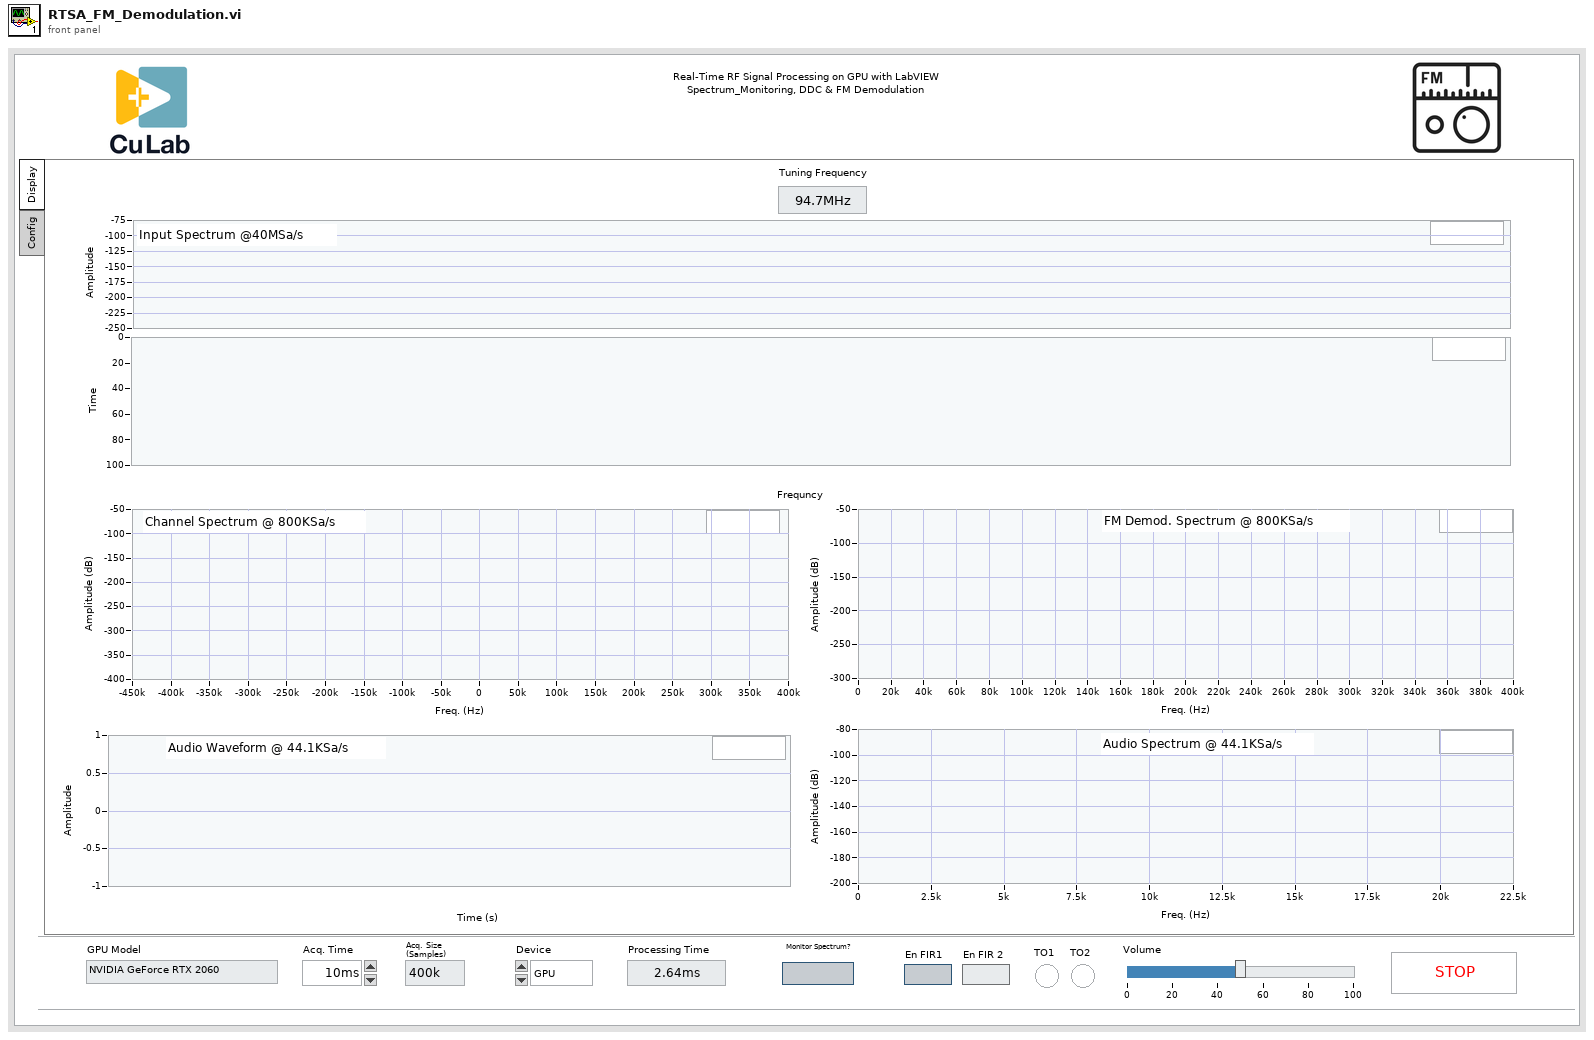
[diagram p1: front panel]
types:
  T1 = cluster{"mean":dbl, "Acq. Time":dbl, "Procesing Loop Time":dbl}
  T2 = enum16{"None ", "Hanning", "Hamming", "Blackman-Harris", "Exact Blackman", "Blackman", "Flat Top", "4 Term B-Harris ", "7 Term B-Harris", "Low Sidelobe", "Blackman Nuttall"}
  T3 = typedef "Sound Data Format.ctl" = cluster{"sample rate (S/s)":dbl, "number of channels":i32, "bits per sample":i32}
  T4 = typedef "Sampling Mode.ctl" = i32
  T5 = typedef "FIR_Config.ctl" = cluster{"filter type":T6, "taps":i32, "high cutoff freq: fh":dbl, "sampling freq: fs":dbl, "low cutoff freq: fl":dbl, "window":T7, "option":enum32{"not scaled", "scaled"}}
  T6 = typedef "NI_AALBase.lvlib/Filter Passband Type.ctl" = enum32{"Lowpass", "Highpass", "Bandpass", "Bandstop"}
  T7 = typedef "NI_AALPro.lvlib/windowTd.ctl" = u32
  T8 = enum16{"open", "open or create", "create or replace", "create", "open (read-only)"}
  T9 = typedef "High Speed Stream-c(dbl,a[.](i8)).lvlib/)Channel.ctl" = refnum<queue>
  T10 = typedef "CuLab.lvlib/Properties.ctl" = cluster{"Device ID":i32, "Name":string}
  T11 = cluster{"alias rejection (dB)":dbl, "normalized bandwidth":dbl}
  T12 = typedef "High Speed Stream-a[.](sgl).lvlib/)Channel.ctl" = refnum<queue>
  T13 = typedef "Sound Output Task ID.ctl" = u32
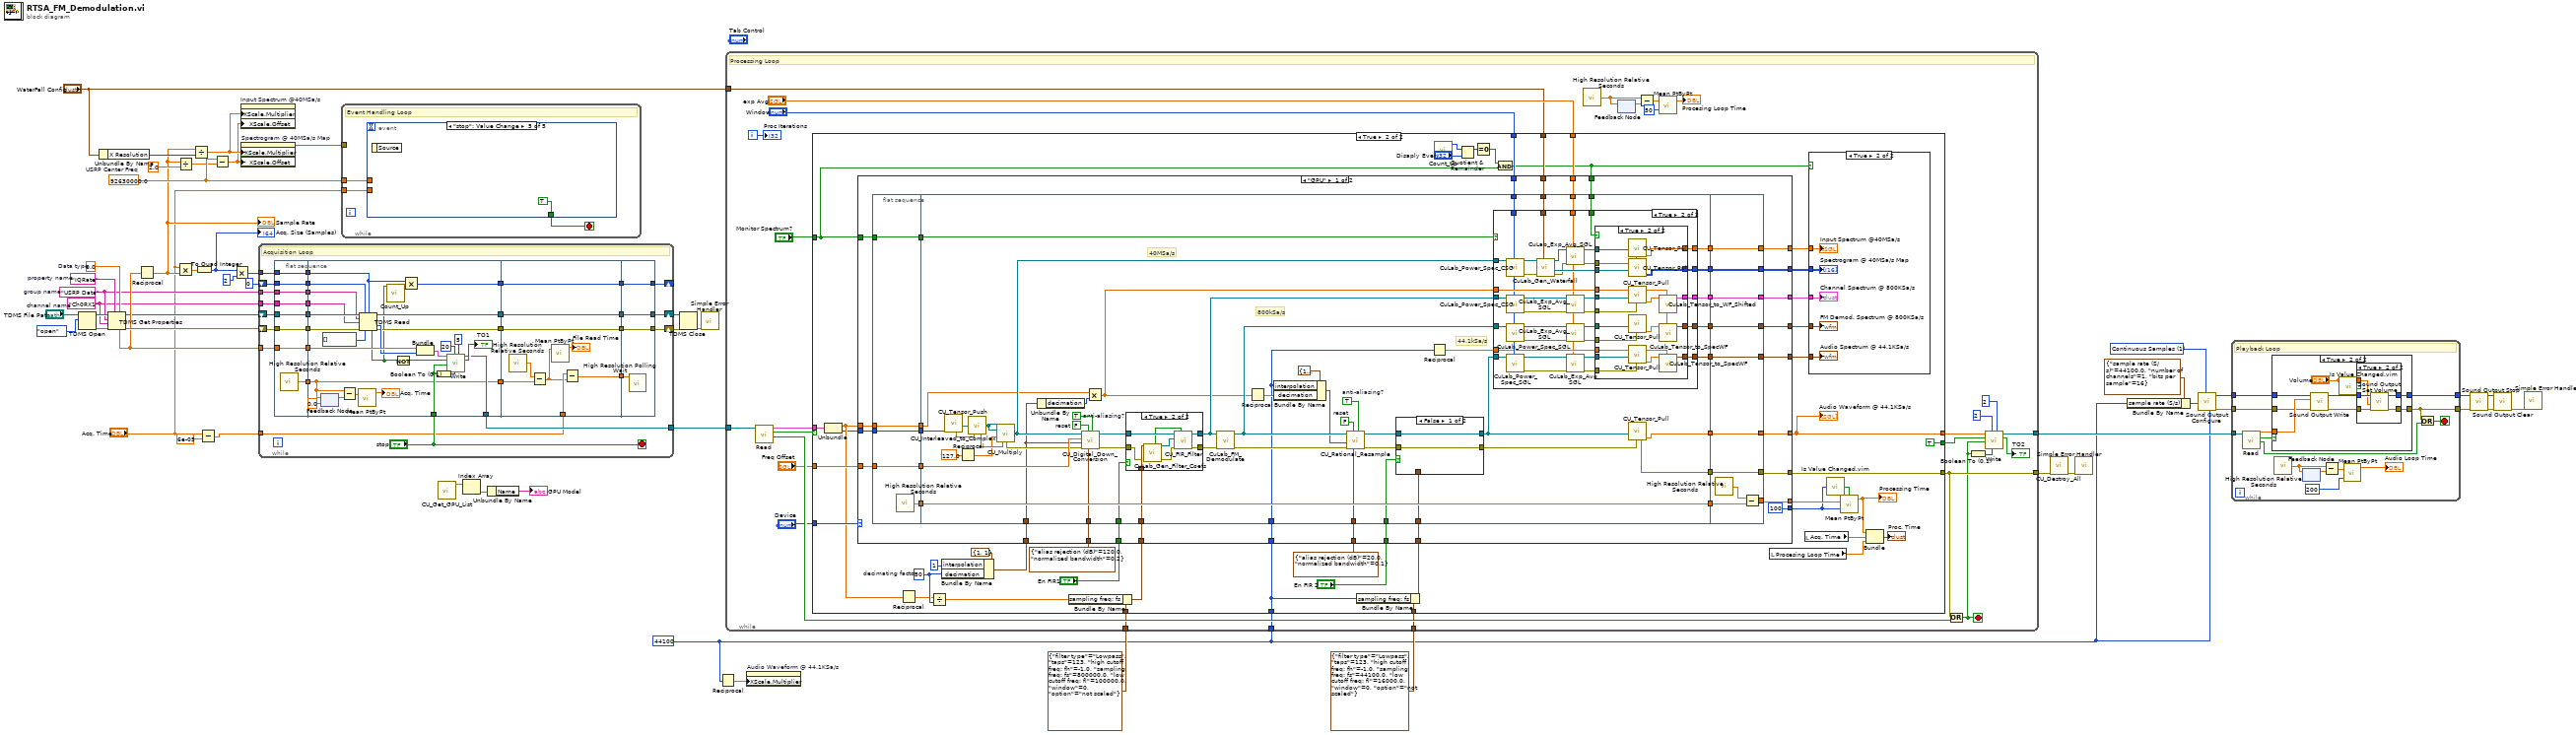
[diagram p0: block diagram]
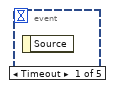
[diagram p2: hidden frame]
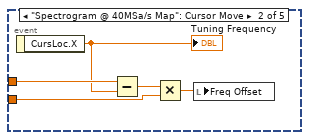
[diagram p3: hidden frame]
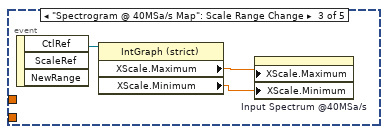
[diagram p4: hidden frame]
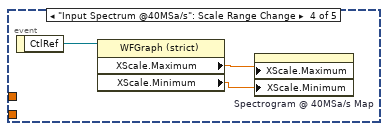
[diagram p5: hidden frame]
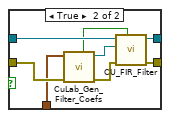
[diagram p8: hidden frame]
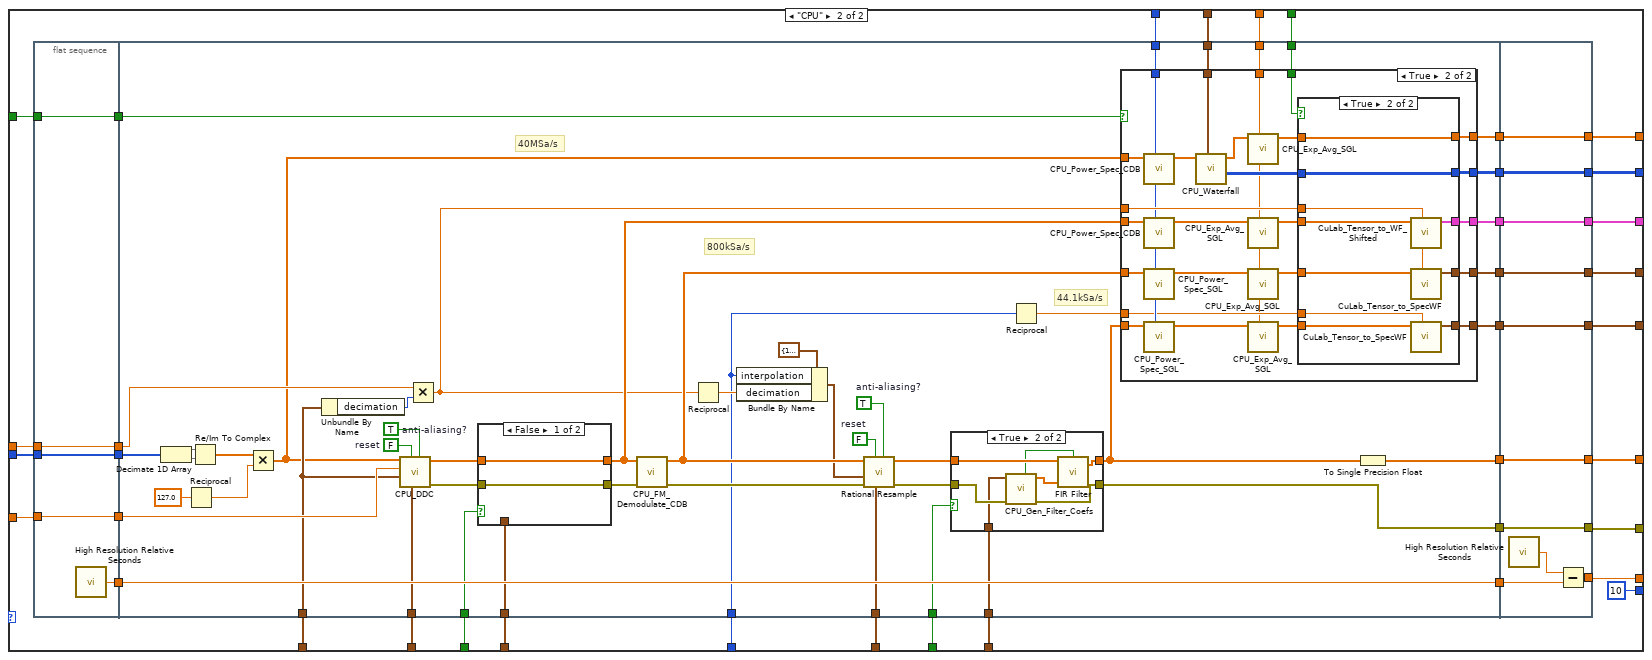
[diagram p11: hidden frame]
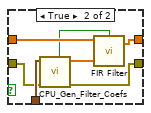
[diagram p12: hidden frame]
diagram:
  w12 = T4 1 items=["Finite Samples", "Continuous Samples"] ("Public Parameters.sample mode")
  w4 = 44100 ("desired sample rate (Hz)")
  w25 = 0.0  # Data type
  w26 = "IQRate"  # property name
  w21 = "Ch0RX1"  # channel name
  w22 = "USRP Data"  # group name
  w43 = 92630000.0  # USRP Center Freq
  n1 = TDMS Open(10:T8."open" ("operation (0:open)"), 11:"TDMS File Path") -> (0:w50:errorcluster, 3:w52:refnum<k34>)  [unwired: 5 in]
  n2 = Unbundle By Name("WaterFall Config") -> ("X Resolution"=w41:i32)
  n3 = TDMS Get Properties(5:w25, 7:w26, 8:w50, 9:w21, 10:w22, 11:w52) -> (0:w35:errorcluster, 3:w23:refnum<k34>, 4:w24:dbl)  [unwired: 3 out]
  n4 = Reciprocal(x=w24) -> (1/x=w36:dbl)
  "Sample Rate" <- w36
  n5 = Multiply(x="Acq. Time", y=w36) -> (x*y=w40:dbl)
  n6 = Divide(x=w36, y=2.0 ("x")) -> (x/y=w42:dbl)
  n7 = Divide(x=w36, y=w41) -> (x/y=w33:dbl)
  n8 = To Quad Integer(1:w40) -> (0:w28:i64)
  "Acq. Size (Samples)" <- w28
  n9 = Subtract(x="Acq. Time", y=6e-05) -> (x-y=w2:dbl)
  n10 = Subtract(x=w43, y=w42) -> (x-y=w32:dbl)
  n11 = Multiply(x=w28, y=i64 2) -> (x*y=w27:i64)
  n12 = property on="Input Spectrum @40MSa/s" class="WFGraph (strict)"("XScale.Multiplier"=w33, "XScale.Offset"=w32) -> ()  [unwired: 2 in, 2 out]
  n13 = property on="Spectrogram @ 40MSa/s Map" class="IntGraph (strict)"("XScale.Multiplier"=w33, "XScale.Offset"=w32) -> (error out=w49:errorcluster)  [unwired: 2 in, 1 out]
  n14 = while {
    tunnel: w24 -> [w78]
    shift-right: [w81] -> w37
    shift-left: w23 -> [w80]
    shift-right: [w69] -> w38
    shift-left: w35 -> [w79]
    tunnel: [w68] -> w34
    tunnel: w2 -> [w53]
    tunnel: w27 -> [w77]
    tunnel: w22 -> [w66]
    tunnel: w21 -> [w65]
    shift-right: [w60] -> _
    shift-left: i64 0 ("offset (0)") -> [w63]
    stop <- "stop" stop-if-true
    # "Acquisition Loop"
    n15 = flat-sequence {
      tunnel: [w89] -> w76
      tunnel: [w88] -> w75
      tunnel: [w87] -> w74
      tunnel: [w86] -> w73
      tunnel: w77 -> [w86]
      tunnel: w78 -> [w87]
      tunnel: w79 -> [w88]
      tunnel: w80 -> [w89]
      tunnel: [w85] -> w67
      tunnel: w66 -> [w85]
      tunnel: w65 -> [w84]
      tunnel: [w84] -> w64
      tunnel: w63 -> [w83]
      tunnel: [w83] -> w62
      tunnel: [w82] -> w54
      tunnel: w76 -> [w106]
      tunnel: w75 -> [w105]
      tunnel: w74 -> [w116]
      tunnel: w73 -> [w97]
      tunnel: [w101] -> w72
      tunnel: [w102] -> w71
      tunnel: "stop" -> [w109]
      tunnel: [w111] -> w68
      tunnel: w67 -> [w100]
      tunnel: w64 -> [w99]
      tunnel: w62 -> [w95]
      tunnel: [w96] -> w61
      tunnel: [w91] -> w55
      tunnel: w54 -> [w91]
      tunnel: w72 -> [w125]
      tunnel: w71 -> [w124]
      tunnel: w61 -> [w123]
      tunnel: [w125] -> w59
      tunnel: [w124] -> w58
      tunnel: [w123] -> w57
      tunnel: [w120] -> w56
      tunnel: w55 -> [w121]
      tunnel: w53 -> [w119]
      tunnel: [w127] -> w60
      tunnel: [w128] -> w69
      tunnel: [w129] -> w81
      tunnel: w59 -> [w129]
      tunnel: w58 -> [w128]
      tunnel: w57 -> [w127]
      tunnel: w56 -> [w126]
      frame #0 {
        n16 = call <vilib>:"High Resolution Relative Seconds.vi"() -> ("relative seconds"=w82:dbl)
      }
      frame #1 {
        n17 = feedback #1(0.0 ("relative seconds")) -> (w94:dbl)
        n18 = feedback-in #1(w91) -> ()
        n19 = Subtract(x=w91, y=w94) -> (x-y=w93:dbl)
        n20 = call <vilib>:"Mean PtByPt.vi"("x"=w93) -> ("mean"=→"Acq. Time":dbl)  [unwired: 3 in, 1 out]
        n21 = TDMS Read(0:w106, 1:w95, 2:w97, 5:w100, 7:w99, 11:w105, 12:i8[] []) -> (4:w101:refnum<k34>, 10:w104:i8[], 14:w98:bool, 15:w102:errorcluster)  [unwired: 1 in, 2 out]
        n22 = call "Count_Up.vi"("Reset?"=w98) -> ("t"=w108:i64)  [unwired: 10 in]
        n23 = Not(x=w98) -> (.not. x?=w103:bool)
        n24 = Multiply(x=w97, y=w108) -> (x*y=w96:i64)
        n25 = Bundle(w116, w104) -> (w115:cluster{dbl, i8[]})  [unwired: 1 in]
        n26 = Boolean To (0,1)(Boolean=w109) -> (0, 1=w110:i16)
        n27 = call <extravilib>:"Write.vi"("timeout in ms (-1)"=5, "abort status (no abort)"=w110, "size (unlimited)"=20, "last element? (F)"=w109, "element valid? (T)"=w103, "element"=w115) -> ("timed out?"=→"TO1":bool, "channel"=w111:T9)  [unwired: 3 in, 1 out]
      }
      frame #2 {
        n28 = call <vilib>:"High Resolution Relative Seconds.vi"() -> ("relative seconds"=w122:dbl)
        n29 = Subtract(x=w122, y=w121) -> (x-y=w117:dbl)
        n30 = call <vilib>:"Mean PtByPt.vi"("x"=w117) -> ("mean"=→"File Read Time":dbl)  [unwired: 3 in, 1 out]
        n31 = Subtract(x=w119, y=w117) -> (x-y=w120:dbl)
      }
      frame #3 {
        n32 = call <vilib>:"High Resolution Polling Wait.vi"("seconds to wait"=w126) -> ()  [unwired: 10 in, 1 out]
      }
    }
  }
  n33 = while {
    tunnel: w49 -> [_]
    tunnel: w43 -> [w131]
    tunnel: "Acq. Time" -> [w130]
    stop <- w132 stop-if-true
    # "Event Handling Loop"
    n34 = event shown="[4] \"stop\": Value Change" {
      selector: _ -> [_ _ _ _ _]
      dyn-events: _ -> [_ _ _ _ _]
      timeout: _ -> [_ _ _ _ _]
      tunnel: [_ _ _ _ TRUE] -> w132
      tunnel: w131 -> [_ w136 _ _ _]
      tunnel: w130 -> [_ w134 _ _ _]
      event Timeout {
        n35 = event-data() -> ()  [unwired: 1 in, 1 out]
      }
      event "Spectrogram @ 40MSa/s Map": Cursor Move {
        n36 = event-data() -> ("CursLoc.X"=w133:dbl)  [unwired: 1 in]
        "Tuning Frequency" <- w133
        n37 = Subtract(x=w136, y=w133) -> (x-y=w135:dbl)
        n38 = Multiply(x=w135, y=w134) -> (x*y=w137:dbl)
        n39 = local write "Freq Offset"(w137) -> ()
      }
      event "Spectrogram @ 40MSa/s Map": Scale Range Change {
        n40 = event-data() -> ("CtlRef"=w140:refnum<vi>)  [unwired: 1 in, 2 out]
        n41 = property class="IntGraph (strict)"(reference=w140) -> ("XScale.Maximum"=w139:dbl, "XScale.Minimum"=w138:dbl)  [unwired: 1 in, 2 out]
        n42 = property on="Input Spectrum @40MSa/s" class="WFGraph (strict)"("XScale.Maximum"=w139, "XScale.Minimum"=w138) -> ()  [unwired: 2 in, 2 out]
      }
      event "Input Spectrum @40MSa/s": Scale Range Change {
        n43 = event-data() -> ("CtlRef"=w143:refnum<vi>)  [unwired: 1 in]
        n44 = property class="WFGraph (strict)"(reference=w143) -> ("XScale.Maximum"=w142:dbl, "XScale.Minimum"=w141:dbl)  [unwired: 1 in, 2 out]
        n45 = property on="Spectrogram @ 40MSa/s Map" class="IntGraph (strict)"("XScale.Maximum"=w142, "XScale.Minimum"=w141) -> ()  [unwired: 2 in, 2 out]
      }
      event "stop": Value Change {
        n46 = event-data() -> ()  [unwired: 1 in, 1 out]
      }
    }
  }
  n47 = call <vilib>:"CU_Get_GPU_List.vi"() -> ("Devices"=w47:T10[])  [unwired: 10 in, 1 out]
  n48 = Index Array(array=w47) -> (element=w46:T10)  [unwired: 1 in]
  n49 = Unbundle By Name(w46) -> ("Name"=→"GPU Model":string)
  n50 = TDMS Close(8:w38, 11:w37) -> (0:w29:errorcluster)  [unwired: 1 out]
  n51 = call <vilib>:"Simple Error Handler.vi"("error in (no error)"=w29) -> ()  [unwired: 4 in, 5 out]
  n52 = Reciprocal(x=w4) -> (1/x=w19:dbl)
  n53 = while {
    tunnel: w34 -> [w161]
    tunnel: [w169] -> w16
    tunnel: "WaterFall Config" -> [w162]
    tunnel: T5 {"filter type"=enum."Lowpass", "taps"=123, "high cutoff freq: fh"=-1.0, "sampling freq: fs"=800000.0, "low cutoff freq: fl"=100000.0, "window"=0, "option"=enum."not scaled"} ("FIR3 Config 15kHz") -> [w155]
    tunnel: T5 {"filter type"=enum."Lowpass", "taps"=123, "high cutoff freq: fh"=-1.0, "sampling freq: fs"=44100.0, "low cutoff freq: fl"=16000.0, "window"=0, "option"=enum."not scaled"} ("FIR3 Config 15kHz") -> [w154]
    tunnel: [w147] -> w15
    tunnel: w4 -> [w145]
    i -> [w172]
    stop <- w146 stop-if-true
    # "Processing Loop"
    n54 = call <extravilib>:"Read.vi"("channel"=w161) -> ("done?"=w170:bool, "element valid?"=w163:bool, "element"=w171:cluster{dbl, i8[]})  [unwired: 6 in, 2 out]
    n55 = case shown="True" w163 {
      tunnel: w171 -> [_ w174]
      tunnel: [_ w184] -> w169
      tunnel: "Device" -> [_ w201]
      tunnel: "Freq Offset" -> [_ w215]
      tunnel: "Monitor Spectrum?" -> [_ w199]
      tunnel: w162 -> [_ w209]
      tunnel: "Window" -> [_ w208]
      tunnel: "exp Avg" -> [_ w207]
      tunnel: w155 -> [_ w181]
      tunnel: w154 -> [_ w180]
      tunnel: [_ w179] -> w149
      tunnel: [_ TRUE] -> w148
      tunnel: w145 -> [_ w177]
      frame False {
      }
      frame True {
        w193 = 50  # decimating factor
        n56 = Unbundle(w174) -> (w175:dbl, w173:i8[])
        n57 = Reciprocal(x=w175) -> (1/x=w190:dbl)
        n58 = Divide(x=w190, y=w193) -> (x/y=w194:dbl)
        n59 = Bundle By Name(cluster=cluster{"interpolation":i32, "decimation":i32} {"interpolation"=1, "decimation"=1} ("resample factor"), "interpolation"=1, "decimation"=w193) -> (w195:cluster{"interpolation":i32, "decimation":i32})
        n60 = Bundle By Name(cluster=w181, "sampling freq: fs"=w194) -> (w192:T5)
        n61 = Bundle By Name(cluster=w180, "sampling freq: fs"=w177) -> (w183:T5)
        n62 = call "Count_Up.vi"() -> ("t"=w176:i64)  [unwired: 11 in]
        n63 = Quotient & Remainder(x=w176, y="Disaply Every") -> (x-y*floor(x/y)=w204:i64)  [unwired: 1 out]
        n64 = Equal To 0?(x=w204) -> (x = 0?=w203:bool)
        n65 = And(x=w203, y=w199) -> (x .and. y?=w188:bool)
        n66 = case shown="\"GPU\"" w201 {
          tunnel: w175 -> [w254 w432]
          tunnel: w183 -> [w253 w431]
          tunnel: [w252 w430] -> w184
          tunnel: [w251 w429] -> w179
          tunnel: [w250 w428] -> w212
          tunnel: [w240 w418] -> w211
          tunnel: w215 -> [w249 w427]
          tunnel: [w241 w419] -> w214
          tunnel: w199 -> [w228 w406]
          tunnel: [w238 w416] -> w213
          tunnel: [100 ("sample length") 10 ("sample length")] -> w185
          tunnel: [w234 w412] -> w210
          tunnel: [w233 w411] -> w206
          tunnel: w209 -> [w231 w409]
          tunnel: w208 -> [w230 w408]
          tunnel: w207 -> [w229 w407]
          tunnel: T11 {"alias rejection (dB)"=20.0, "normalized bandwidth"=0.1} ("FIR filter specifications") -> [w226 w404]
          tunnel: w192 -> [w225 w403]
          tunnel: T11 {"alias rejection (dB)"=120.0, "normalized bandwidth"=0.2} ("FIR filter specifications") -> [w224 w402]
          tunnel: w195 -> [w223 w401]
          tunnel: w173 -> [w222 w400]
          tunnel: "En FIR1" -> [w220 w398]
          tunnel: "En FIR 2" -> [w219 w397]
          tunnel: w188 -> [w218 w396]
          tunnel: w177 -> [w217 w395]
          frame "GPU" {
            n67 = flat-sequence {
              tunnel: w249 -> [w258]
              tunnel: w254 -> [w259]
              tunnel: [w259] -> w245
              tunnel: [w258] -> w244
              tunnel: [w257] -> w242
              tunnel: w228 -> [w256]
              tunnel: [w256] -> w227
              tunnel: w222 -> [w255]
              tunnel: [w255] -> w221
              tunnel: w253 -> [w285]
              tunnel: [w266] -> w248
              tunnel: [w269] -> w247
              tunnel: [w311] -> w246
              tunnel: w245 -> [w274]
              tunnel: w244 -> [w310]
              tunnel: [w299] -> w243
              tunnel: w242 -> [w299]
              tunnel: [w298] -> w239
              tunnel: [w297] -> w237
              tunnel: [w295] -> w235
              tunnel: [w294] -> w232
              tunnel: w231 -> [w293]
              tunnel: w230 -> [w292]
              tunnel: w229 -> [w291]
              tunnel: w227 -> [w289]
              tunnel: w226 -> [w286]
              tunnel: w225 -> [w278]
              tunnel: w224 -> [w276]
              tunnel: w223 -> [w273]
              tunnel: w221 -> [w275]
              tunnel: w220 -> [w271]
              tunnel: w219 -> [w270]
              tunnel: w218 -> [w265]
              tunnel: w217 -> [w260]
              tunnel: [w392] -> w250
              tunnel: [w393] -> w251
              tunnel: [w394] -> w252
              tunnel: w248 -> [w394]
              tunnel: w247 -> [w393]
              tunnel: w246 -> [w392]
              tunnel: w243 -> [w389]
              tunnel: [w391] -> w241
              tunnel: [w388] -> w240
              tunnel: w239 -> [w388]
              tunnel: [w387] -> w238
              tunnel: w237 -> [w387]
              tunnel: w235 -> [w386]
              tunnel: [w386] -> w234
              tunnel: [w385] -> w233
              tunnel: w232 -> [w385]
              frame #0 {
                n68 = call <vilib>:"High Resolution Relative Seconds.vi"() -> ("relative seconds"=w257:dbl)
              }
              frame #1 {
                w263 = FALSE  # reset
                w262 = FALSE  # reset
                w280 = TRUE  # anti-aliasing?
                w306 = TRUE  # anti-aliasing?
                # "44.1kSa/s"
                # "800kSa/s"
                # "40MSa/s"
                n69 = call-poly <vilib>:"CU_Tensor_Push.vi"("T1D_I8_Data"=w275) -> ("T1D_I8 out"=w277:refnum<class "T1D_I8.lvclass">, "error out"=w304:errorcluster)  [unwired: 9 in]
                n70 = Reciprocal(x=127.0 ("relative seconds")) -> (1/x=w264:dbl)
                n71 = call-poly <vilib>:"CU_Interleaved_to_Complex.vi"("x"=w277, "error in (no error)"=w304) -> ("Dest out"=w300:refnum<class "T1D_CSG.lvclass">, "error out"=w302:errorcluster)  [unwired: 12 in]
                n72 = call-poly <vilib>:"CU_Multiply.vi"("Dest in"=w300, "x"=w300, "y"=w264, "error in (no error)"=w302) -> ("Dest out"=w288:refnum<class "T1D_CSG.lvclass">, "error out"=w303:errorcluster)  [unwired: 10 in]
                n73 = Unbundle By Name(w273) -> ("decimation"=w272:i32)
                n74 = call-poly <vilib>:"CU_Digital_Down_Conversion.vi"("anti-aliasing?"=w280, "FIR filter specifications"=w276, "reset"=w263, "error in"=w303, "resample factor"=w273, "shift frequency"=w310, "X"=w288) -> ("error out"=w282:errorcluster, "Y"=w284:refnum<class "T1D_CSG.lvclass">)  [unwired: 3 in]
                n75 = Multiply(x=w274, y=w272) -> (x*y=w279:dbl)
                n76 = case shown="True" w271 {
                  tunnel: w284 -> [w313 w321]
                  tunnel: [w313 w320] -> w283
                  tunnel: w282 -> [w312 w314]
                  tunnel: [w312 w319] -> w281
                  tunnel: w278 -> [_ w318]
                  frame False {
                  }
                  frame True {
                    n77 = call "CuLab_Gen_Filter_Coefs.vi"("error in (no error)"=w314, "FIR Config"=w318) -> ("error out"=w315:errorcluster, "Coefs"=w317:refnum<class "T1D_SGL.lvclass">, "FIR Init/Continue"=w316:bool)  [unwired: 7 in]
                    n78 = call-poly <vilib>:"CU_FIR_Filter.vi"("init/cont (init:F)"=w316, "error in (no error)"=w315, "FIR Coefficients"=w317, "X"=w321) -> ("error out"=w319:errorcluster, "Filtered X"=w320:refnum<class "T1D_CSG.lvclass">)  [unwired: 6 in]
                  }
                }
                n79 = call "CuLab_FM_Demodulate.vi"("error in (no error)"=w281, "Signal In"=w283) -> ("error out"=w309:errorcluster, "FM Demod Out"=w296:refnum<class "T1D_SGL.lvclass">)  [unwired: 8 in]
                n80 = Reciprocal(x=w279) -> (1/x=w307:dbl)
                n81 = Bundle By Name(cluster=cluster{"interpolation":i32, "decimation":i32} {"interpolation"=1, "decimation"=100} ("resample factor"), "interpolation"=w260, "decimation"=w307) -> (w290:cluster{"interpolation":i32, "decimation":i32})
                n82 = call-poly <vilib>:"CU_Rational_Resample.vi"("anti-aliasing?"=w306, "FIR filter specifications"=w286, "reset"=w262, "error in (no error)"=w309, "resample factor"=w290, "X"=w296) -> ("error out"=w305:errorcluster, "Y"=w287:refnum<class "T1D_SGL.lvclass">)  [unwired: 3 in, 1 out]
                n83 = case shown="False" w270 {
                  tunnel: w305 -> [w322 w331]
                  tunnel: [w322 w330] -> w267
                  tunnel: [w323 w329] -> w268
                  tunnel: w287 -> [w323 w328]
                  tunnel: w285 -> [_ w327]
                  frame False {
                  }
                  frame True {
                    n84 = call "CuLab_Gen_Filter_Coefs.vi"("error in (no error)"=w331, "FIR Config"=w327) -> ("error out"=w325:errorcluster, "Coefs"=w324:refnum<class "T1D_SGL.lvclass">, "FIR Init/Continue"=w326:bool)  [unwired: 7 in]
                    n85 = call-poly <vilib>:"CU_FIR_Filter.vi"("init/cont (init:F)"=w326, "error in (no error)"=w325, "FIR Coefficients"=w324, "X"=w328) -> ("error out"=w330:errorcluster, "Filtered X"=w329:refnum<class "T1D_SGL.lvclass">)  [unwired: 6 in]
                  }
                }
                n86 = Reciprocal(x=w260) -> (1/x=w261:dbl)
                n87 = case shown="True" w289 {
                  tunnel: [_ w358] -> w311
                  tunnel: w296 -> [_ w363]
                  tunnel: w283 -> [_ w364]
                  tunnel: w279 -> [_ w352]
                  tunnel: [_ w350] -> w298
                  tunnel: w261 -> [_ w343]
                  tunnel: w268 -> [_ w365]
                  tunnel: [_ w351] -> w297
                  tunnel: w288 -> [_ w362]
                  tunnel: w293 -> [_ w361]
                  tunnel: [_ w347] -> w295
                  tunnel: [_ w348] -> w294
                  tunnel: w292 -> [_ w344]
                  tunnel: w291 -> [_ w342]
                  tunnel: w265 -> [_ w341]
                  frame False {
                  }
                  frame True {
                    n88 = call "CuLab_Power_Spec_CSG.vi"("window"=w344, "T1D_CSG in"=w362) -> ("error out"=w339:errorcluster, "log(x)"=w357:refnum<class "T1D_SGL.lvclass">)  [unwired: 8 in]
                    n89 = call "CuLab_Power_Spec_CSG.vi"("window"=w344, "T1D_CSG in"=w364) -> ("error out"=w338:errorcluster, "log(x)"=w360:refnum<class "T1D_SGL.lvclass">)  [unwired: 8 in]
                    n90 = call "CuLab_Power_Spec_SGL.vi"("window"=w344, "T1D_SGL in"=w363) -> ("error out"=w337:errorcluster, "Pwr Spec"=w353:refnum<class "T1D_SGL.lvclass">)  [unwired: 8 in]
                    n91 = call "CuLab_Power_Spec_SGL.vi"("window"=w344, "T1D_SGL in"=w365) -> ("error out"=w336:errorcluster, "Pwr Spec"=w354:refnum<class "T1D_SGL.lvclass">)  [unwired: 8 in]
                    n92 = call "CuLab_Gen_Waterfall.vi"("WaterFall Config"=w361, "error in (no error)"=w339, "Y"=w357) -> ("error IO"=w340:errorcluster, "WaterFall"=w349:refnum<class "T2D_I16.lvclass">, "WF Decimated"=w346:refnum<class "T1D_SGL.lvclass">)  [unwired: 6 in]
                    n93 = call "CuLab_Exp_Avg_SGL.vi"("exp Avg Factor"=w342, "error in (no error)"=w340, "T1D_SGL in"=w346) -> ("error out"=w335:errorcluster, "T1D_SGL out"=w345:refnum<class "T1D_SGL.lvclass">)  [unwired: 7 in]
                    n94 = call "CuLab_Exp_Avg_SGL.vi"("exp Avg Factor"=w342, "error in (no error)"=w338, "T1D_SGL in"=w360) -> ("error out"=w334:errorcluster, "T1D_SGL out"=w359:refnum<class "T1D_SGL.lvclass">)  [unwired: 7 in]
                    n95 = call "CuLab_Exp_Avg_SGL.vi"("exp Avg Factor"=w342, "error in (no error)"=w337, "T1D_SGL in"=w353) -> ("error out"=w333:errorcluster, "T1D_SGL out"=w356:refnum<class "T1D_SGL.lvclass">)  [unwired: 7 in]
                    n96 = call "CuLab_Exp_Avg_SGL.vi"("exp Avg Factor"=w342, "error in (no error)"=w336, "T1D_SGL in"=w354) -> ("error out"=w332:errorcluster, "T1D_SGL out"=w355:refnum<class "T1D_SGL.lvclass">)  [unwired: 7 in]
                    n97 = case shown="True" w341 {
                      tunnel: w359 -> [_ w384]
                      tunnel: [_ w383] -> w358
                      tunnel: w356 -> [_ w382]
                      tunnel: w355 -> [_ w381]
                      tunnel: w352 -> [_ w380]
                      tunnel: [_ w379] -> w351
                      tunnel: [_ w378] -> w350
                      tunnel: w349 -> [_ w377]
                      tunnel: [_ w367] -> w348
                      tunnel: [_ w376] -> w347
                      tunnel: w345 -> [_ w366]
                      tunnel: w343 -> [_ w375]
                      tunnel: w335 -> [_ w371]
                      tunnel: w334 -> [_ w370]
                      tunnel: w333 -> [_ w369]
                      tunnel: w332 -> [_ w368]
                      frame False {
                      }
                      frame True {
                        n98 = call-poly <vilib>:"CU_Tensor_Pull.vi"("error in (no error)"=w371, "T1D_SGL in"=w366) -> ("Dest out"=w367:sgl[])  [unwired: 7 in, 2 out]
                        n99 = call-poly <vilib>:"CU_Tensor_Pull.vi"("T2D_I16 in"=w377) -> ("Dest out"=w376:i16[][])  [unwired: 8 in, 2 out]
                        n100 = call-poly <vilib>:"CU_Tensor_Pull.vi"("error in (no error)"=w370, "T1D_SGL in"=w384) -> ("Dest out"=w372:sgl[])  [unwired: 7 in, 2 out]
                        n101 = call-poly <vilib>:"CU_Tensor_Pull.vi"("error in (no error)"=w369, "T1D_SGL in"=w382) -> ("Dest out"=w373:sgl[])  [unwired: 7 in, 2 out]
                        n102 = call-poly <vilib>:"CU_Tensor_Pull.vi"("error in (no error)"=w368, "T1D_SGL in"=w381) -> ("Dest out"=w374:sgl[])  [unwired: 7 in, 2 out]
                        n103 = call "CuLab_Tensor_to_WF_Shifted.vi"("dt"=w380, "Y"=w372) -> ("WF"=w383:cluster{dbl, dbl, "Dest out":sgl[]})  [unwired: 9 in]
                        n104 = call "CuLab_Tensor_to_SpecWF.vi"("dt"=w380, "Y"=w373) -> ("Spectrum WF"=w378:waveform(sgl))  [unwired: 9 in]
                        n105 = call "CuLab_Tensor_to_SpecWF.vi"("dt"=w375, "Y"=w374) -> ("Spectrum WF"=w379:waveform(sgl))  [unwired: 9 in]
                      }
                    }
                  }
                }
                n106 = call-poly <vilib>:"CU_Tensor_Pull.vi"("error in (no error)"=w267, "T1D_SGL in"=w268) -> ("Dest out"=w269:sgl[], "error out"=w266:errorcluster)  [unwired: 7 in, 1 out]
              }
              frame #2 {
                n107 = call <vilib>:"High Resolution Relative Seconds.vi"() -> ("relative seconds"=w390:dbl)
                n108 = Subtract(x=w390, y=w389) -> (x-y=w391:dbl)
              }
            }
          }
          frame "CPU" {
            n109 = flat-sequence {
              tunnel: w427 -> [w436]
              tunnel: w432 -> [w437]
              tunnel: [w437] -> w423
              tunnel: [w436] -> w422
              tunnel: [w435] -> w420
              tunnel: w406 -> [w434]
              tunnel: [w434] -> w405
              tunnel: w400 -> [w433]
              tunnel: [w433] -> w399
              tunnel: w431 -> [w465]
              tunnel: [w441] -> w426
              tunnel: [w440] -> w425
              tunnel: [w486] -> w424
              tunnel: w423 -> [w456]
              tunnel: w422 -> [w485]
              tunnel: [w478] -> w421
              tunnel: w420 -> [w478]
              tunnel: [w477] -> w417
              tunnel: [w476] -> w415
              tunnel: [w474] -> w413
              tunnel: [w473] -> w410
              tunnel: w409 -> [w472]
              tunnel: w408 -> [w471]
              tunnel: w407 -> [w470]
              tunnel: w405 -> [w468]
              tunnel: w404 -> [w466]
              tunnel: w403 -> [w458]
              tunnel: w402 -> [w457]
              tunnel: w401 -> [w455]
              tunnel: w399 -> [w444]
              tunnel: w398 -> [w453]
              tunnel: w397 -> [w452]
              tunnel: w396 -> [w450]
              tunnel: w395 -> [w438]
              tunnel: [w547] -> w428
              tunnel: [w548] -> w429
              tunnel: [w549] -> w430
              tunnel: w426 -> [w549]
              tunnel: w425 -> [w548]
              tunnel: w424 -> [w547]
              tunnel: w421 -> [w544]
              tunnel: [w546] -> w419
              tunnel: [w543] -> w418
              tunnel: w417 -> [w543]
              tunnel: [w542] -> w416
              tunnel: w415 -> [w542]
              tunnel: w413 -> [w541]
              tunnel: [w541] -> w412
              tunnel: [w540] -> w411
              tunnel: w410 -> [w540]
              frame #0 {
                n110 = call <vilib>:"High Resolution Relative Seconds.vi"() -> ("relative seconds"=w435:dbl)
              }
              frame #1 {
                w448 = FALSE  # reset
                w449 = FALSE  # reset
                w460 = TRUE  # anti-aliasing?
                w481 = TRUE  # anti-aliasing?
                # "44.1kSa/s"
                # "800kSa/s"
                # "40MSa/s"
                n111 = Decimate 1D Array(w444) -> (w446:i8[], w447:i8[])
                n112 = Reciprocal(x=127.0 ("relative seconds")) -> (1/x=w443:dbl)
                n113 = Re/Im To Complex(1:w447, 2:w446) -> (0:w445:cdb[])
                n114 = Multiply(x=w445, y=w443) -> (x*y=w442:cdb[])
                n115 = Unbundle By Name(w455) -> ("decimation"=w454:i32)
                n116 = call "CPU_DDC.vi"("anti-aliasing?"=w460, "FIR filter specifications"=w457, "reset"=w449, "resample factor"=w455, "Freq Offset"=w485, "Array"=w442) -> ("error out"=w462:errorcluster, "Y"=w464:cdb[])  [unwired: 4 in]
                n117 = Multiply(x=w456, y=w454) -> (x*y=w459:dbl)
                n118 = case shown="False" w453 {
                  tunnel: w464 -> [w488 w495]
                  tunnel: [w488 w494] -> w463
                  tunnel: w462 -> [w487 w490]
                  tunnel: [w487 w489] -> w461
                  tunnel: w458 -> [_ w493]
                  frame False {
                  }
                  frame True {
                    n119 = call "CPU_Gen_Filter_Coefs.vi"("error in"=w490, "FIR Config"=w493) -> ("error out"=w489:errorcluster, "FIR_Coeffs"=w492:dbl[], "FIR Init/Continue"=w491:bool)  [unwired: 7 in]
                    n120 = call-poly <vilib>:"FIR Filter.vi"("init/cont (init:F)"=w491, "FIR Coefficients"=w492, "X"=w495) -> ("Filtered X"=w494:cdb[])  [unwired: 1 in, 1 out]
                  }
                }
                n121 = call "CPU_FM_Demodulate_CDB.vi"("error in (no error)"=w461, "1D_CDB in"=w463) -> ("error out"=w484:errorcluster, "1D_DBL out"=w475:dbl[])  [unwired: 7 in, 1 out]
                n122 = Reciprocal(x=w459) -> (1/x=w482:dbl)
                n123 = Bundle By Name(cluster=cluster{"interpolation":i32, "decimation":i32} {"interpolation"=1, "decimation"=100} ("resample factor"), "interpolation"=w438, "decimation"=w482) -> (w469:cluster{"interpolation":i32, "decimation":i32})
                n124 = call-poly <vilib>:"Rational Resample.vi"("anti-aliasing?"=w481, "FIR filter specifications"=w466, "reset"=w448, "error in (no error)"=w484, "resample factor"=w469, "X"=w475) -> ("error out"=w480:errorcluster, "Y"=w467:dbl[])  [unwired: 3 in, 1 out]
                n125 = case shown="True" w452 {
                  tunnel: w480 -> [w496 w504]
                  tunnel: [w496 w498] -> w441
                  tunnel: [w497 w503] -> w451
                  tunnel: w467 -> [w497 w502]
                  tunnel: w465 -> [_ w501]
                  frame False {
                  }
                  frame True {
                    n126 = call "CPU_Gen_Filter_Coefs.vi"("error in"=w504, "FIR Config"=w501) -> ("error out"=w498:errorcluster, "FIR_Coeffs"=w499:dbl[], "FIR Init/Continue"=w500:bool)  [unwired: 7 in]
                    n127 = call-poly <vilib>:"FIR Filter.vi"("init/cont (init:F)"=w500, "FIR Coefficients"=w499, "X"=w502) -> ("Filtered X"=w503:dbl[])  [unwired: 1 in, 1 out]
                  }
                }
                n128 = Reciprocal(x=w438) -> (1/x=w439:dbl)
                n129 = case shown="True" w468 {
                  tunnel: [_ w523] -> w486
                  tunnel: w475 -> [_ w527]
                  tunnel: w463 -> [_ w528]
                  tunnel: w459 -> [_ w519]
                  tunnel: [_ w517] -> w477
                  tunnel: w439 -> [_ w510]
                  tunnel: w451 -> [_ w529]
                  tunnel: [_ w518] -> w476
                  tunnel: w442 -> [_ w526]
                  tunnel: w472 -> [_ w525]
                  tunnel: [_ w514] -> w474
                  tunnel: [_ w515] -> w473
                  tunnel: w471 -> [_ w511]
                  tunnel: w470 -> [_ w509]
                  tunnel: w450 -> [_ w508]
                  frame False {
                  }
                  frame True {
                    n130 = call "CPU_Power_Spec_CDB.vi"("window"=w511, "Signal"=w526) -> ("Spectrum (no Avg)"=w522:dbl[])  [unwired: 9 in]
                    n131 = call "CPU_Power_Spec_CDB.vi"("window"=w511, "Signal"=w528) -> ("Spectrum (no Avg)"=w507:dbl[])  [unwired: 9 in]
                    n132 = call "CPU_Power_Spec_SGL.vi"("window"=w511, "Signa"=w527) -> ("x*y"=w505:sgl[])  [unwired: 9 in]
                    n133 = call "CPU_Power_Spec_SGL.vi"("window"=w511, "Signa"=w529) -> ("x*y"=w506:sgl[])  [unwired: 9 in]
                    n134 = call "CPU_Waterfall.vi"("Config"=w525, "Spectrum"=w522) -> ("DownSampled Waterfall"=w516:i16[][], "DownSampled Spectrum"=w513:sgl[])  [unwired: 8 in]
                    n135 = call "CPU_Exp_Avg_SGL.vi"("exp Avg Factor"=w509, "Data"=w513) -> ("Exp Out"=w512:sgl[])  [unwired: 9 in]
                    n136 = call "CPU_Exp_Avg_SGL.vi"("exp Avg Factor"=w509, "Data"=w507) -> ("Exp Out"=w524:sgl[])  [unwired: 9 in]
                    n137 = call "CPU_Exp_Avg_SGL.vi"("exp Avg Factor"=w509, "Data"=w505) -> ("Exp Out"=w521:sgl[])  [unwired: 9 in]
                    n138 = call "CPU_Exp_Avg_SGL.vi"("exp Avg Factor"=w509, "Data"=w506) -> ("Exp Out"=w520:sgl[])  [unwired: 9 in]
                    n139 = case shown="True" w508 {
                      tunnel: w524 -> [_ w532]
                      tunnel: [_ w539] -> w523
                      tunnel: w521 -> [_ w531]
                      tunnel: w520 -> [_ w530]
                      tunnel: w519 -> [_ w538]
                      tunnel: [_ w537] -> w518
                      tunnel: [_ w536] -> w517
                      tunnel: w516 -> [_ w535]
                      tunnel: [_ w533] -> w515
                      tunnel: [_ w535] -> w514
                      tunnel: w512 -> [_ w533]
                      tunnel: w510 -> [_ w534]
                      frame False {
                      }
                      frame True {
                        n140 = call "CuLab_Tensor_to_WF_Shifted.vi"("dt"=w538, "Y"=w532) -> ("WF"=w539:cluster{dbl, dbl, "Dest out":sgl[]})  [unwired: 9 in]
                        n141 = call "CuLab_Tensor_to_SpecWF.vi"("dt"=w538, "Y"=w531) -> ("Spectrum WF"=w536:waveform(sgl))  [unwired: 9 in]
                        n142 = call "CuLab_Tensor_to_SpecWF.vi"("dt"=w534, "Y"=w530) -> ("Spectrum WF"=w537:waveform(sgl))  [unwired: 9 in]
                      }
                    }
                  }
                }
                n143 = To Single Precision Float(number=w451) -> (single precision float=w440:sgl[])
              }
              frame #2 {
                n144 = call <vilib>:"High Resolution Relative Seconds.vi"() -> ("relative seconds"=w545:dbl)
                n145 = Subtract(x=w545, y=w544) -> (x-y=w546:dbl)
              }
            }
          }
        }
        "Audio Waveform @ 44.1KSa/s" <- w179
        n146 = local read "Procesing Loop Time"() -> (w182:dbl)
        n147 = local read "Acq. Time"() -> (w186:dbl)
        n148 = case shown="True" w188 {
          tunnel: w213 -> [_ w554]
          tunnel: w212 -> [_ w553]
          tunnel: w211 -> [_ w552]
          tunnel: w210 -> [_ w551]
          tunnel: w206 -> [_ w550]
          frame False {
          }
          frame True {
            "FM Demod. Spectrum @ 800KSa/s" <- w552
            "Channel Spectrum @ 800KSa/s" <- w553
            "Audio Spectrum @ 44.1KSa/s" <- w554
            "Input Spectrum @40MSa/s" <- w550
            "Spectrogram @ 40MSa/s Map" <- w551
          }
        }
        n149 = call "Is Value Changed.vim"("value"=w185) -> ("changed or first call?"=w200:bool)
        n150 = call <vilib>:"Mean PtByPt.vi"("x"=w214, "sample length"=w185, "initialize"=w200) -> ("mean"=w202:dbl)  [unwired: 1 in, 1 out]
        "Processing Time" <- w202
        n151 = Bundle("mean"=w202, "Acq. Time"=w186, "Procesing Loop Time"=w182) -> (→"Proc. Time":T1)  [unwired: 1 in]
      }
    }
    n152 = call <vilib>:"High Resolution Relative Seconds.vi"() -> ("relative seconds"=w159:dbl)
    n153 = feedback #2() -> (w160:dbl)  [unwired: 1 in]
    n154 = feedback-in #2(w159) -> ()
    n155 = Subtract(x=w159, y=w160) -> (x-y=w157:dbl)
    n156 = call <vilib>:"Mean PtByPt.vi"("x"=w157, "sample length"=50) -> ("mean"=→"Procesing Loop Time":dbl)  [unwired: 2 in, 1 out]
    n157 = Or(x=w169, y=w170) -> (x .or. y?=w146:bool)
    n158 = Boolean To (0,1)(Boolean=w146) -> (0, 1=w153:i16)
    n159 = call <extravilib>:"Write.vi"("timeout in ms (-1)"=2, "abort status (no abort)"=w153, "size (unlimited)"=2, "last element? (F)"=w146, "element valid? (T)"=w148, "element"=w149) -> ("timed out?"=→"TO2":bool, "channel"=w147:T12)  [unwired: 3 in, 1 out]
    "Proc Iterations" <- w172
  }
  n160 = property on="Audio Waveform @ 44.1KSa/s" class="WFGraph (strict)"("XScale.Multiplier"=w19) -> ()  [unwired: 2 in, 2 out]
  n161 = call <vilib>:"CU_Destroy_All.vi"("error in"=w16) -> ("error out"=w48:errorcluster)  [unwired: 10 in]
  n162 = call <vilib>:"Simple Error Handler.vi"("error in (no error)"=w48) -> ()  [unwired: 4 in, 5 out]
  n163 = Bundle By Name(cluster=T3 {"sample rate (S/s)"=44100.0, "number of channels"=1, "bits per sample"=16} ("Public Parameters.sound format"), "sample rate (S/s)"=w4) -> (w5:T3)
  n164 = call <vilib>:"Sound Output Configure.vi"("number of samples/ch"=w4, "sample mode"=w12, "sound format"=w5) -> ("error out"=w7:errorcluster, "task ID"=w11:T13)  [unwired: 4 in, 3 out]
  n165 = while {
    tunnel: w15 -> [w568]
    tunnel: [w565] -> w13
    tunnel: w11 -> [w564]
    tunnel: [w557] -> w8
    tunnel: w7 -> [w556]
    stop <- w567 stop-if-true
    # "Playback Loop"
    n166 = call <extravilib>:"Read.vi"("channel"=w568) -> ("done?"=w566:bool, "element valid?"=w563:bool, "element"=w559:sgl[])  [unwired: 6 in, 2 out]
    n167 = case shown="True" w563 {
      tunnel: [w570 w579] -> w565
      tunnel: w564 -> [w570 w578]
      tunnel: w559 -> [_ w577]
      tunnel: [w569 w576] -> w557
      tunnel: w556 -> [w569 w575]
      frame False {
      }
      frame True {
        n168 = call-poly <vilib>:"Sound Output Write.vi"("error in (no error)"=w575, "data"=w577, "task ID"=w578) -> ("error out"=w571:errorcluster, "task ID out"=w572:T13)  [unwired: 1 in, 6 out]
        n169 = call "Is Value Changed.vim"("value"="Volume") -> ("changed or first call?"=w573:bool)
        n170 = case shown="True" w573 {
          tunnel: [w581 w585] -> w579
          tunnel: w572 -> [w581 w586]
          tunnel: w571 -> [w580 w584]
          tunnel: "Volume" -> [_ w582]
          tunnel: [w580 w583] -> w576
          frame False {
          }
          frame True {
            n171 = call-poly <vilib>:"Sound Output Set Volume.vi"("error in (no error)"=w584, "volume"=w582, "task ID"=w586) -> ("error out"=w583:errorcluster, "task ID out"=w585:T13)  [unwired: 7 in]
          }
        }
      }
    }
    n172 = call <vilib>:"High Resolution Relative Seconds.vi"() -> ("relative seconds"=w561:dbl)
    n173 = feedback #3() -> (w562:dbl)  [unwired: 1 in]
    n174 = feedback-in #3(w561) -> ()
    n175 = Subtract(x=w561, y=w562) -> (x-y=w560:dbl)
    n176 = call <vilib>:"Mean PtByPt.vi"("x"=w560, "sample length"=200) -> ("mean"=→"Audio Loop Time":dbl)  [unwired: 2 in, 1 out]
    n177 = Or(x=w557, y=w566) -> (x .or. y?=w567:bool)
  }
  n178 = call <vilib>:"Sound Output Stop.vi"("error in (no error)"=w8, "task ID"=w13) -> ("error out"=w14:errorcluster, "task ID out"=w10:T13)  [unwired: 8 in]
  n179 = call <vilib>:"Sound Output Clear.vi"("error in (no error)"=w14, "task ID"=w10) -> ("error out"=w6:errorcluster)  [unwired: 9 in]
  n180 = call <vilib>:"Simple Error Handler.vi"("error in (no error)"=w6) -> ()  [unwired: 4 in, 5 out]
